vi "KB-laser dealwith.vi"(0 "Image  input":T1(plugin-control), 1 "Image  input  copy":T1(plugin-control), 3 "Src Data 过滤0":dbl[][](array[numeric]), 4 "Src Data 过滤3.2":dbl[][](array[numeric]), 5 "Row Select Laser":string(combo)="Item4", 6 "Param List Laser Input":string[][](table), 7 "y":dbl=200.0 format="%#_13g", 8 "数值 2":dbl=0.5 format="%#_13g", 9 "raoto1":dbl=0.8 format="%#_13g") -> (11 "外环3D":dbl[][](array[numeric]), 12 "内外3D":dbl[][](array[numeric]), 13 "内环3D":dbl[][](array[numeric]), 14 "Result Array":string[](array[string]), 15 "Image Baser":T1(plugin-control), 19 "Image Baser 2":T1(plugin-control))   [LabVIEW 2015]
uses:
  <vilib>/vision/Measure.llb/Edge Options.ctl
  <vilib>/vision/Measure.llb/Edge Polarity.ctl
panel:
  out "同心度":dbl
  out "Row Select Laser 2":string(combo)="Item4"
  out "x-y":dbl
  out "矩形ROS new":string[](array[string])
  out "元素":T2 {"Contours"."Type" items=["No Selection", "Point", "Line", "Rectangle", "Oval", "Polygon", "Freehand Region", "Annulus", "Unused2", "Unused3", "Broken Line", "Freehand Line", "Rotated Rectangle"]}
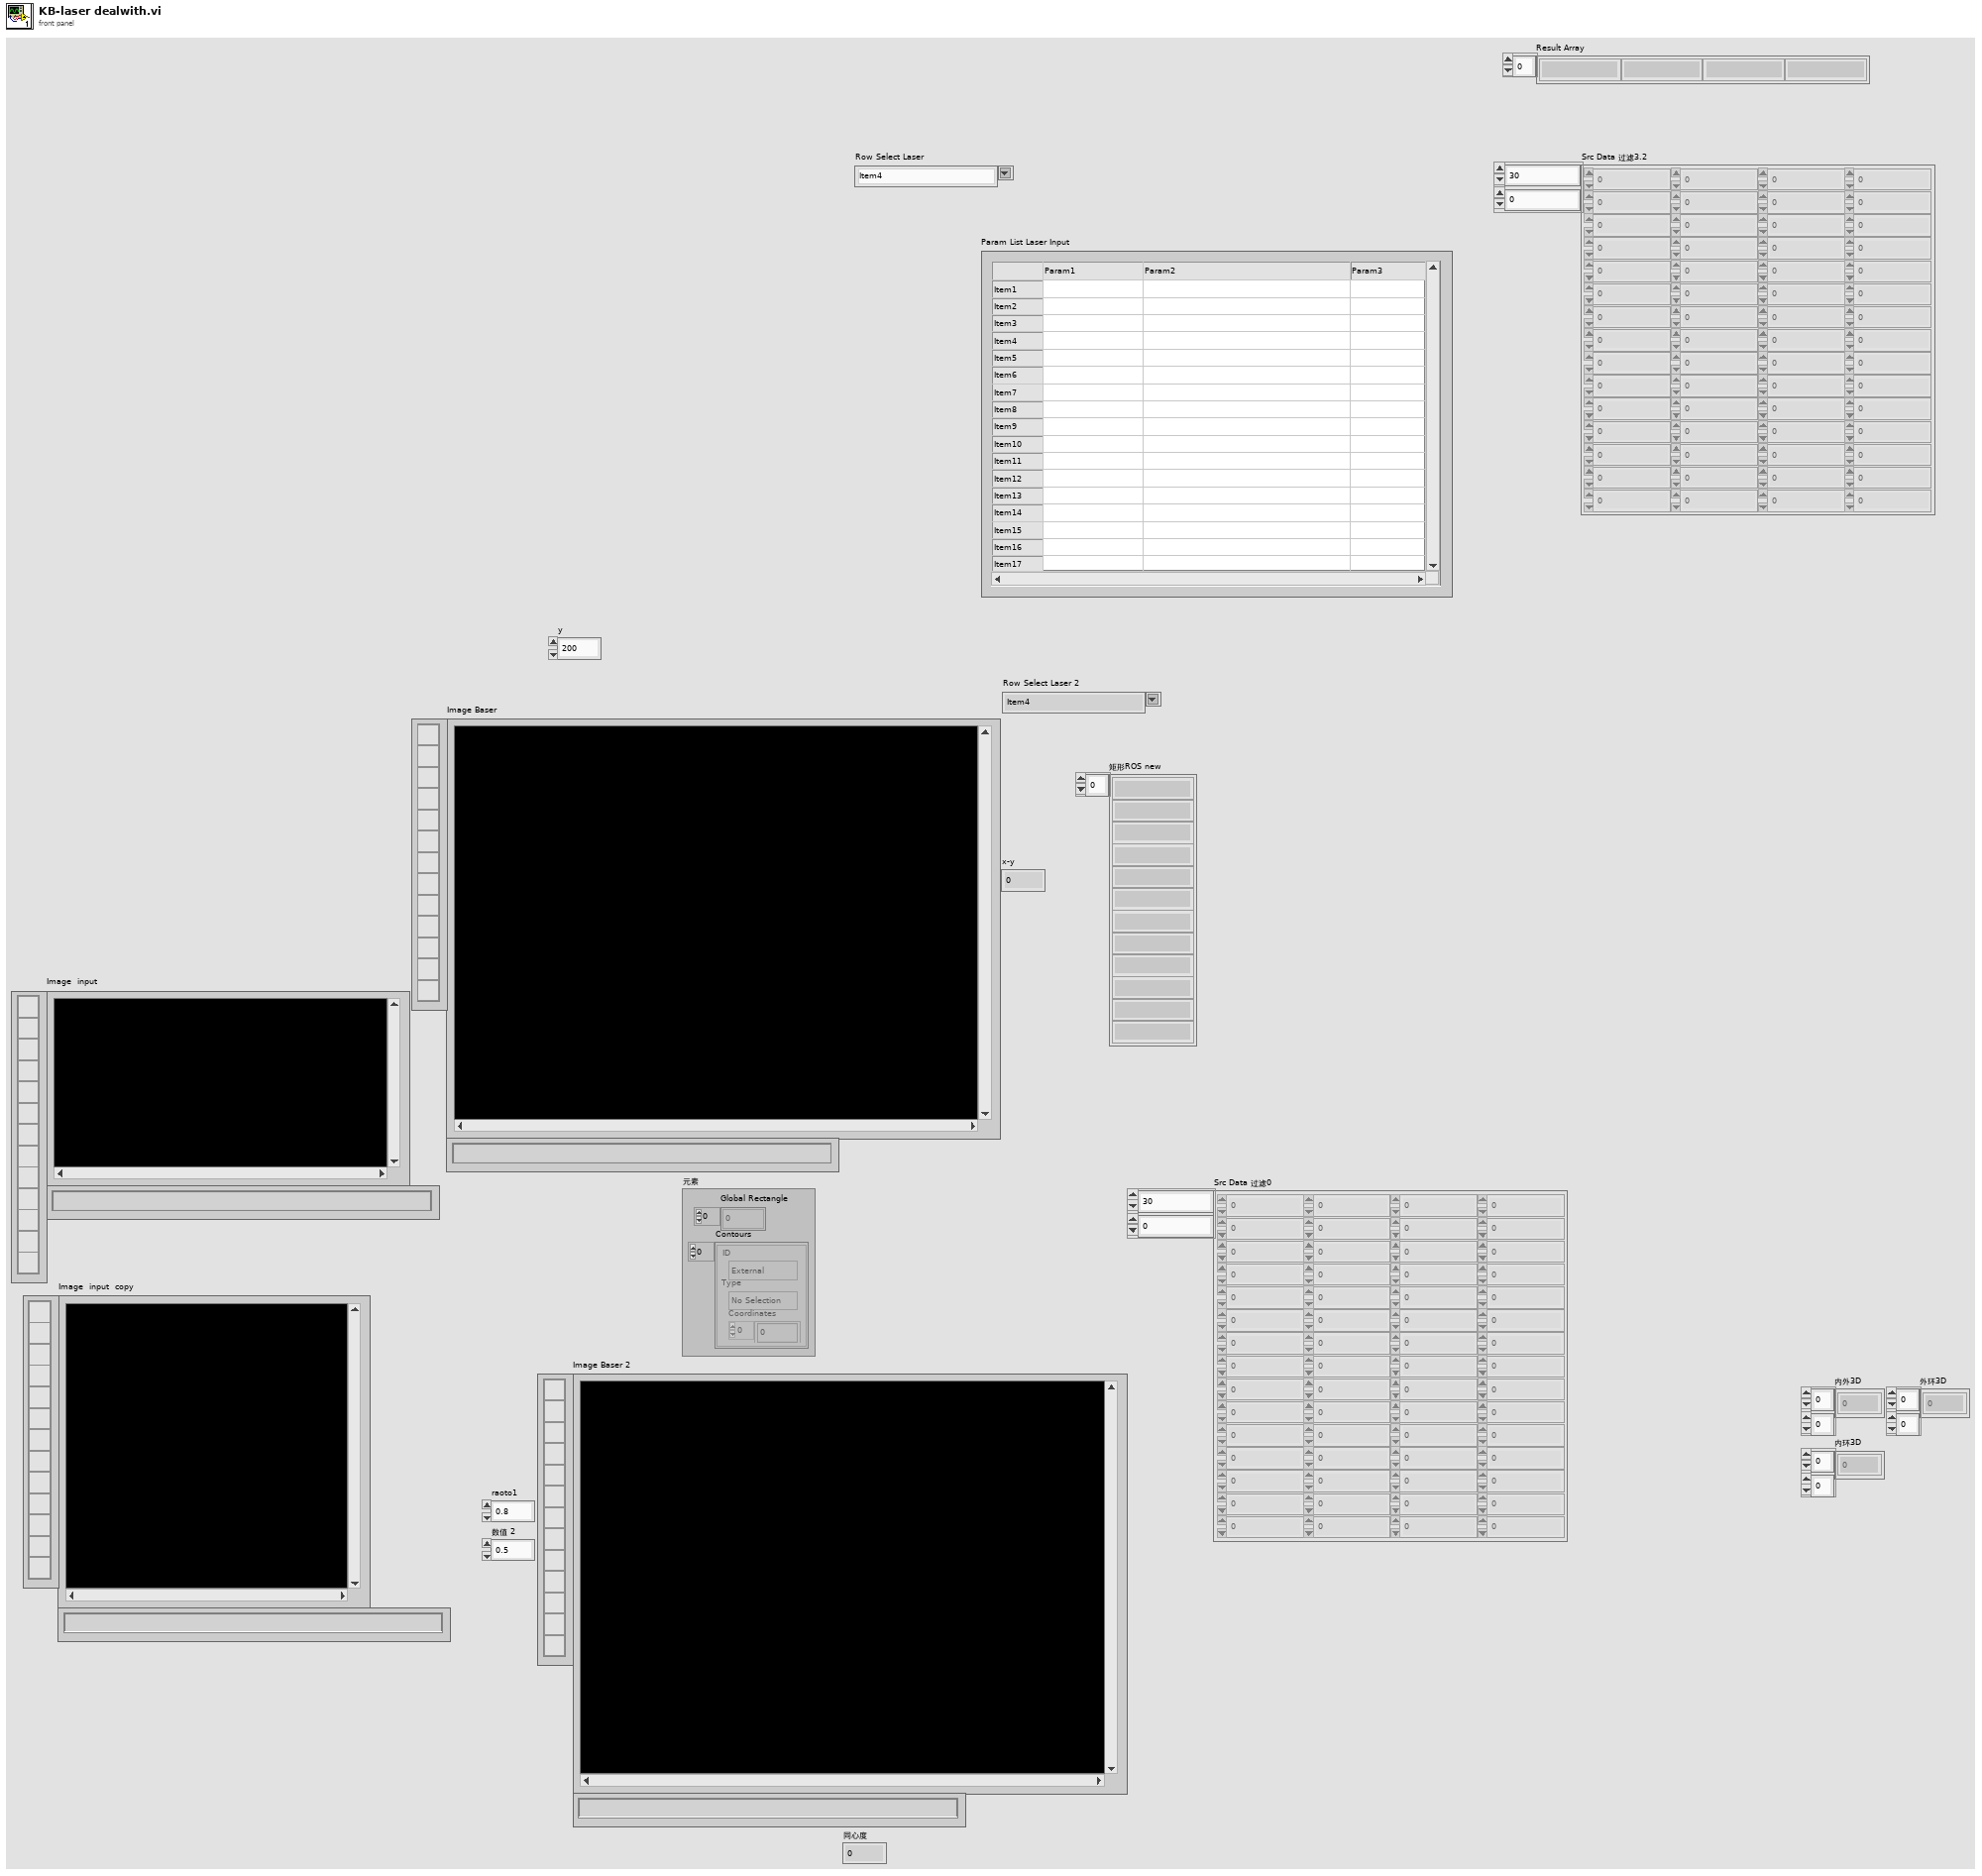
[diagram p1: front panel]
types:
  T1 = typedef "IMAQ Image.ctl" = refnum<image>
  T2 = typedef "ROI Descriptor" = cluster{"Global Rectangle":i32[], "Contours":cluster{"ID":enum32{"External", "Internal"}, "Type":u32, "Coordinates":i32[]}[]}
  T3 = typedef "Edge Options.ctl" = cluster{"Edge Polarity":T4, "Kernel Size":u32, "Width":u32, "Minimum Edge Strength":sgl, "Interpolation Type":enum32{"Zero Order", "Bilinear", "Quadratic", "Cubic", "Bilinear Fixed"}, "Data Processing Method":enum32{"Average", "Median"}}
  T4 = typedef "Edge Polarity.ctl" = u32
  T5 = cluster{"Search  Direction":u32, "Edge Options":T3, "Show Search Area":bool, "Show Search Lines":bool, "Show Edges Found":bool, "Show Result":bool, "Search Area Color":u32, "Search Lines Color":u32, "Edge Locations Color":u32, "Result Color":u32, "Overlay Group Name":string}
  T6 = cluster{"Center (Pixels)":cluster{"X":sgl, "Y":sgl}, "Radius (Pixels)":dbl, "Center (Real-World)":cluster{"X":sgl, "Y":sgl}, "Radius (Real-World)":dbl, "Roundness (Real-World)":dbl, "Average Strength":dbl, "Average SNR (dB)":dbl}
  T7 = typedef "IMAQ GM Match Report.ctl" = cluster{"Position":cluster{"x":sgl, "y":sgl}, "Angle":sgl, "Scale":sgl, "Score":sgl, "Bounding Box":cluster{"x":sgl, "y":sgl}[], "Contrast Reversed":bool, "Occlusion %":sgl, "Template Target Curve Score":sgl, "Target Template Curve Score":sgl, "Correlation Score":sgl}
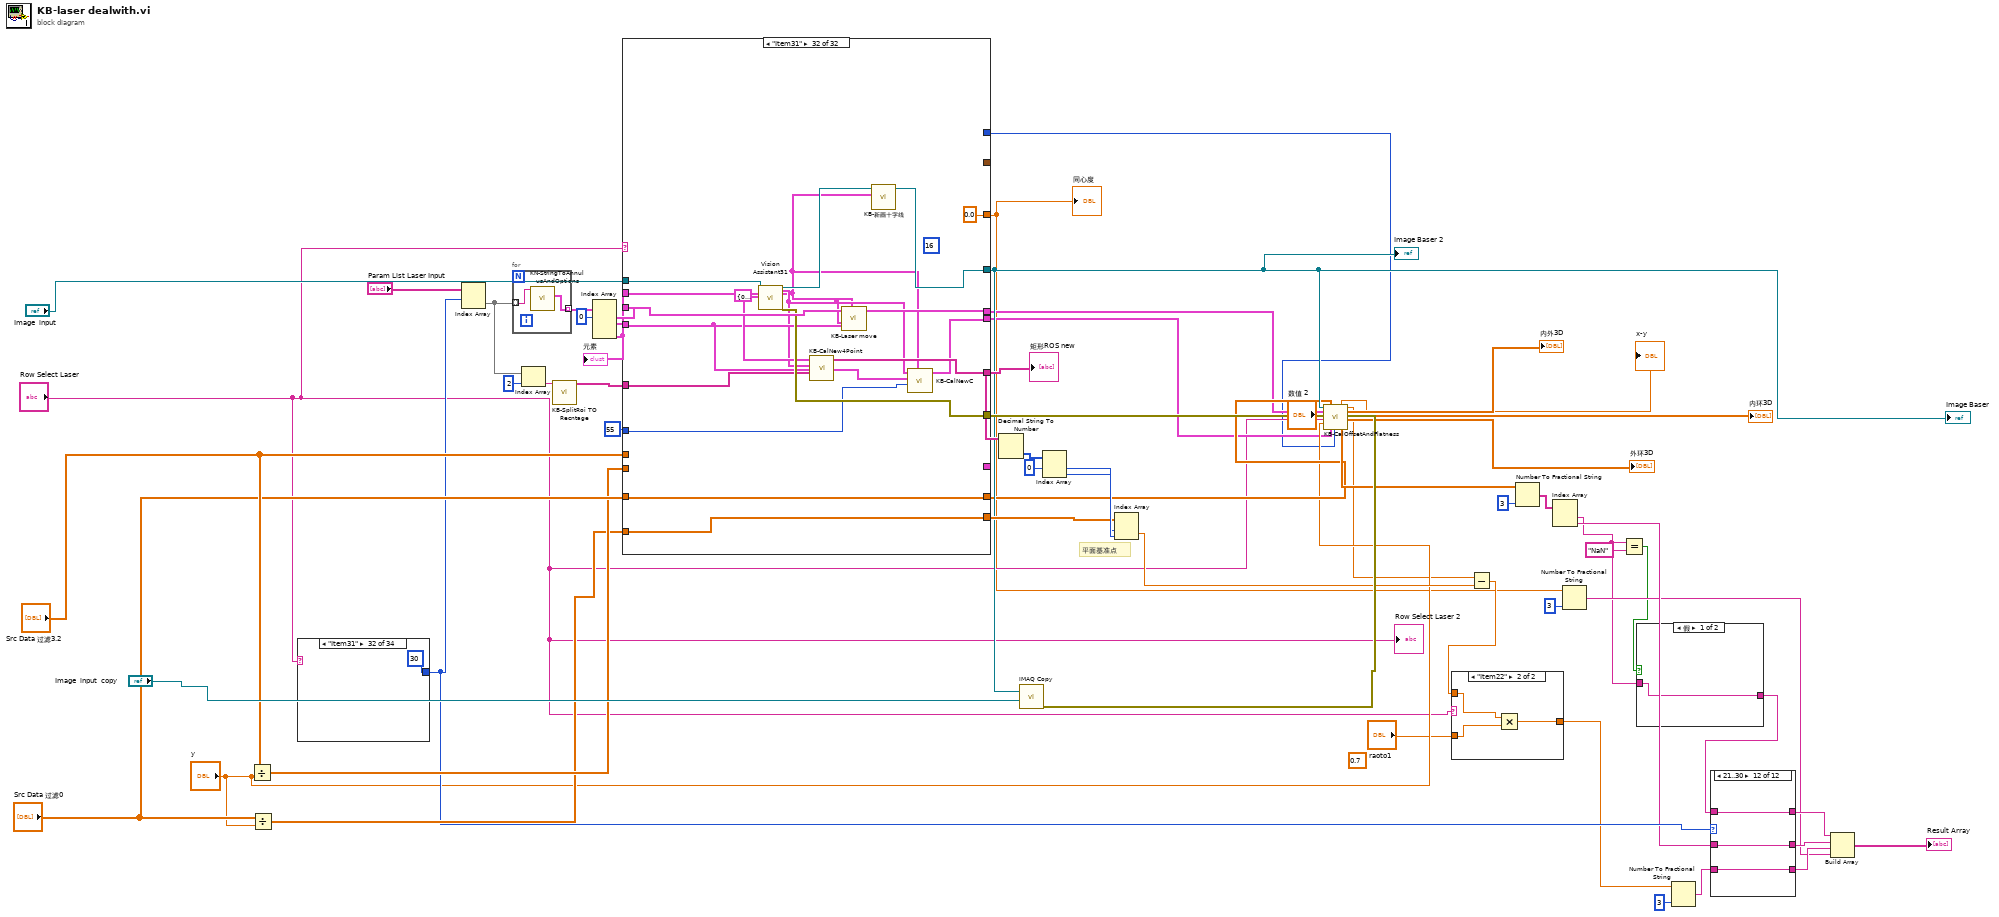
[diagram p0: block diagram]
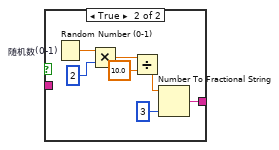
[diagram p2: hidden frame]
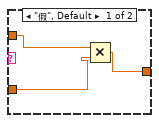
[diagram p3: hidden frame]
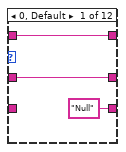
[diagram p4: hidden frame]
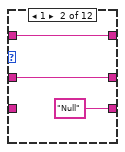
[diagram p5: hidden frame]
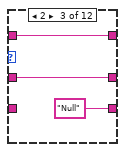
[diagram p6: hidden frame]
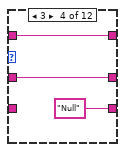
[diagram p7: hidden frame]
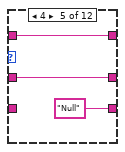
[diagram p8: hidden frame]
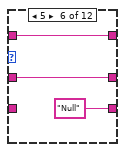
[diagram p9: hidden frame]
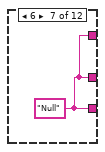
[diagram p10: hidden frame]
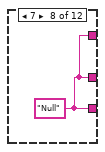
[diagram p11: hidden frame]
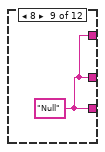
[diagram p12: hidden frame]
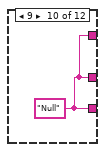
[diagram p13: hidden frame]
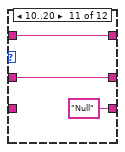
[diagram p14: hidden frame]
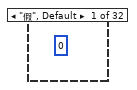
[diagram p15: hidden frame]
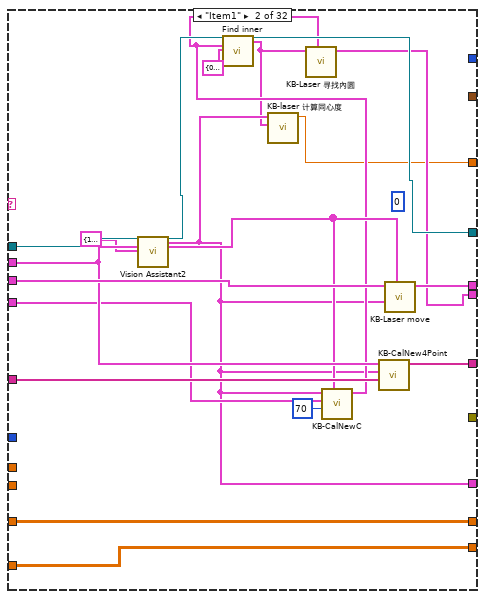
[diagram p16: hidden frame]
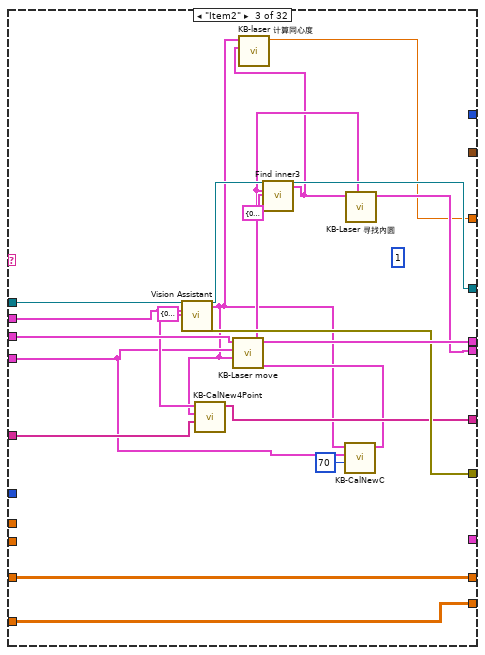
[diagram p17: hidden frame]
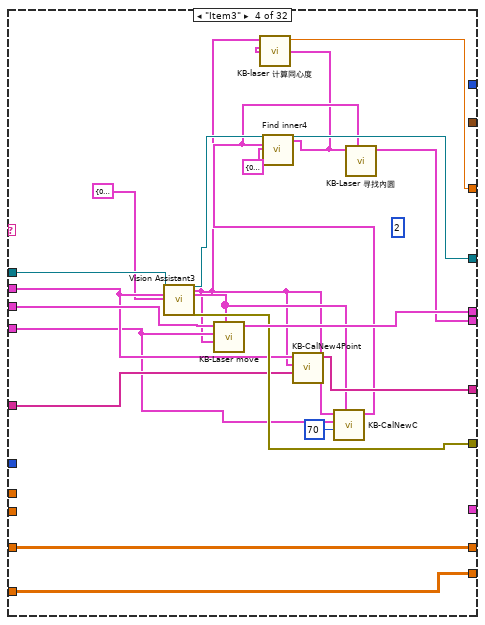
[diagram p18: hidden frame]
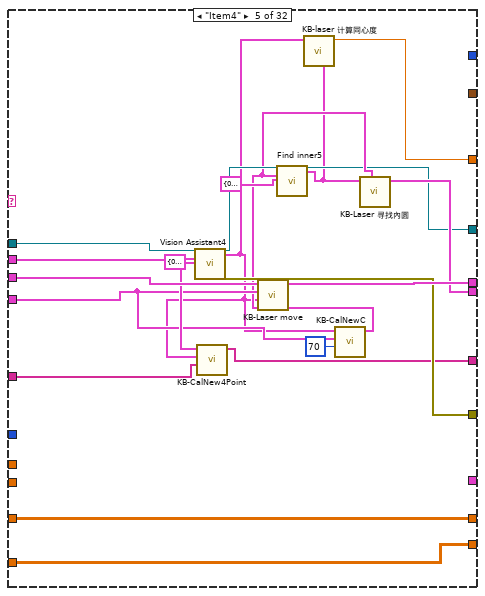
[diagram p19: hidden frame]
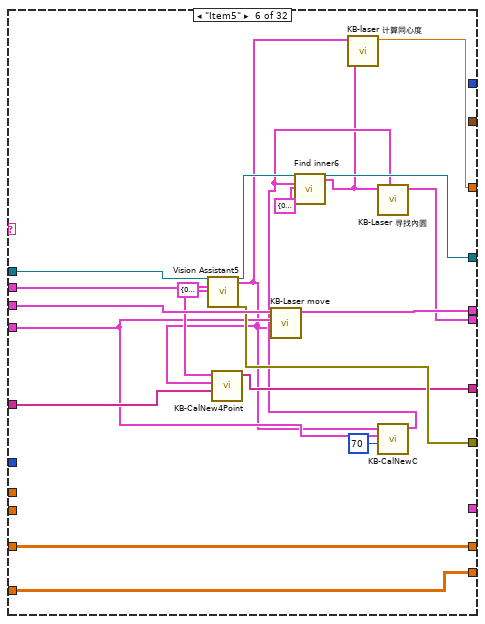
[diagram p20: hidden frame]
diagram:
  (unwired) 0.7 ("y")
  # "平面基准点"
  n1 = Divide(x="Src Data 过滤3.2", y="y") -> (x/y=w43:dbl[][])
  n2 = Divide(x="Src Data 过滤0", y="y") -> (x/y=w42:dbl[][])
  n3 = case shown="\"Item31\"" "Row Select Laser" {
    tunnel: [0 0 1 2 3 4 5 6 7 8 9 10 11 12 13 14 15 16 17 18 19 20 21 22 23 24 25 26 27 28 29 30 31 32] -> w41
    frame "假", Default {
    }
    frame "Item1" {
    }
    frame "Item2" {
    }
    frame "Item3" {
    }
    frame "Item4" {
    }
    frame "Item5" {
    }
    frame "Item6" {
    }
    frame "Item7" {
    }
    frame "Item8" {
    }
    frame "Item9" {
    }
    frame "Item10" {
    }
    frame "Item11" {
    }
    frame "Item12" {
    }
    frame "Item13" {
    }
    frame "Item14" {
    }
    frame "Item15" {
    }
    frame "Item16" {
    }
    frame "Item17" {
    }
    frame "Item18" {
    }
    frame "Item19" {
    }
    frame "Item20" {
    }
    frame "Item21" {
    }
    frame "Item22" {
    }
    frame "Item23" {
    }
    frame "Item24" {
    }
    frame "Item25" {
    }
    frame "Item26" {
    }
    frame "Item27" {
    }
    frame "Item28" {
    }
    frame "Item29" {
    }
    frame "Item30" {
    }
    frame "Item31" {
    }
    frame "Item32" {
    }
    frame "Item33" {
    }
  }
  n4 = Index Array(array="Param List Laser Input", index (row)=w41) -> (element=w54:string[])  [unwired: 1 in]
  n5 = for {
    tunnel: w54 -> [w95] mode=indexing
    tunnel: [w94] -> w58 mode=indexing
    n6 = call "KN-StringToAnnulusAndOptions.vi"("String"=w95) -> ("ROI Descriptor"=w94:T2)  [unwired: 5 in, 5 out]
  }
  n7 = Index Array(array=w54, index=2 ("索引")) -> (element=w52:string)
  n8 = call "KB-SplitRoi TO Recntage.vi"("String 2"=w52) -> ("数组"=w47:string[])  [unwired: 10 in]
  n9 = Index Array(array=w58, index #1=0 ("索引")) -> (element #1=w50:T2, element #2=w49:T2, element #4=w45:T2)  [unwired: 3 in, 1 out]
  "元素" <- w45
  n10 = case shown="\"Item31\"" "Row Select Laser" {
    tunnel: [_ w103 w122 w142 w160 w183 w203 w219 w233 w250 w266 w282 w301 w321 w337 w359 w377 w395 w417 w436 w455 w474 w492 w504 w521 w538 w555 w572 w589 w606 w625 w642] -> w24
    tunnel: "Image  input" -> [_ w115 w135 w156 w176 w196 w215 w229 w243 w259 w275 w294 w314 w328 w352 w372 w391 w410 w429 w448 w467 w486 w494 w517 w534 w551 w568 w585 w592 w619 w637 w655]
    tunnel: w45 -> [_ w112 w131 w152 w172 w192 w212 w226 w240 w256 w272 w291 w311 w327 w349 w369 w388 w407 w426 w445 w464 w483 w493 w514 w531 w548 w565 w582 w600 w616 w634 w651]
    tunnel: w50 -> [_ w114 w134 w155 w175 w195 w214 w228 w242 w258 w274 w293 w313 w333 w351 w371 w390 w409 w428 w447 w466 w485 w502 w516 w533 w550 w567 w584 w602 w618 w636 w654]
    tunnel: w49 -> [_ w102 w128 w149 w169 w189 w209 w223 w237 w249 w265 w288 w308 w329 w346 w366 w385 w404 w423 w442 w461 w480 w499 w511 w528 w545 w562 w579 w597 w613 w631 w648]
    tunnel: [_ w113 w133 w154 w174 w194 w213 w227 w241 w257 w273 w292 w312 w332 w350 w370 w389 w408 w427 w446 w465 w484 w501 w515 w532 w549 w566 w583 w601 w617 w635 w653] -> w22
    tunnel: [_ w100 w120 w140 w162 w181 w201 w222 w236 w248 w264 w280 w299 w319 w339 w357 w378 w397 w415 w434 w453 w472 w498 w510 w527 w544 w561 w578 w596 w612 w630 w647] -> w20
    tunnel: [_ _ w132 w153 w173 w193 _ _ _ _ _ _ _ _ _ _ _ _ _ _ _ _ _ _ _ _ _ _ _ _ _ w652] -> w48
    tunnel: w47 -> [_ w110 w130 w151 w171 w191 w211 w225 w239 w254 w270 w290 w310 w331 w348 w368 w387 w406 w425 w444 w463 w482 w497 w513 w530 w547 w564 w581 w599 w615 w633 w650]
    tunnel: [_ w111 w129 w150 w170 w190 w210 w224 w238 w253 w269 w289 w309 w330 w347 w367 w386 w405 w424 w443 w462 w481 w500 w512 w529 w546 w563 w580 w598 w614 w632 w649] -> w33
    tunnel: "Src Data 过滤3.2" -> [_ _ _ _ _ _ _ _ _ _ _ _ _ _ _ _ _ _ _ _ _ _ _ _ _ _ _ _ _ _ _ _]
    tunnel: "Src Data 过滤0" -> [_ w108 w126 w147 w168 w188 w208 w221 w235 w247 w263 w287 w307 w326 w344 w364 w384 w403 w422 w441 w460 w479 w496 w509 w526 w543 w560 w577 w595 w611 w629 w646]
    tunnel: [_ w108 w126 w147 w168 w188 w208 w221 w235 w247 w263 w287 w307 w326 w344 w364 w384 w403 w422 w441 w460 w479 w496 w509 w526 w543 w560 w577 w595 w611 w629 w646] -> w23
    tunnel: [_ w109 w127 w148 w167 w187 w207 w220 w234 w246 w262 w286 w306 w325 w345 w365 w383 w402 w421 w440 w459 w478 w495 w508 w525 w542 w559 w576 w594 w610 w628 w645] -> w25
    tunnel: w43 -> [_ _ _ _ _ _ _ _ _ _ _ _ _ _ _ _ _ _ _ _ _ _ _ _ _ _ _ _ _ _ _ _]
    tunnel: w42 -> [_ w109 w127 w148 w167 w187 w207 w220 w234 w246 w262 w286 w306 w325 w345 w365 w383 w402 w421 w440 w459 w478 w495 w508 w525 w542 w559 w576 w594 w610 w628 w645]
    tunnel: [_ w98 _ _ _ _ _ _ _ _ _ _ _ _ _ _ _ _ _ _ _ _ _ _ _ _ _ _ _ _ _ _] -> _
    tunnel: 55 ("Outer Radius") -> [_ _ _ _ _ _ _ w217 w231 w245 w261 _ _ _ _ _ _ _ _ _ _ _ _ w506 w523 w540 w557 w574 w591 w608 w627 w640]
    tunnel: [_ _ _ _ _ _ _ _ _ _ _ _ _ _ _ _ _ _ _ _ _ _ _ _ _ _ _ _ _ _ w622 _] -> _
    tunnel: [_ w96 w116 w136 w157 w177 w197 0.0 ("Radius (Real-World)") 0.0 ("Radius (Real-World)") 0.0 ("Radius (Real-World)") 0.0 ("Radius (Real-World)") w276 w295 w315 w334 w353 w373 w392 w411 w430 w449 w468 0.0 ("Radius (Real-World)") 0.0 ("Radius (Real-World)") 0.0 ("Radius (Real-World)") 0.0 ("Radius (Real-World)") 0.0 ("Radius (Real-World)") 0.0 ("Radius (Real-World)") 0.0 ("Radius (Real-World)") 0.0 ("Radius (Real-World)") 0.0 ("Radius (Real-World)") 0.0 ("Radius (Real-World)")] -> w8
    tunnel: [_ _ _ _ _ _ _ _ _ _ _ _ _ _ _ _ _ _ _ _ _ _ 22 _ _ _ _ _ _ _ _ _] -> w10
    frame "假", Default {
      (unwired) 0
    }
    frame "Item1" {
      (unwired) 0
      n11 = call "Vision Assistant2"("Image In"=w115, "ROI Descriptor (Find Circular Edge 1)"=w112, "Options (Find Circular Edge 1)"=T5 {"Search  Direction"=1, "Edge Options"={"Edge Polarity"=2, "Kernel Size"=3, "Width"=3, "Minimum Edge Strength"=38.0, "Interpolation Type"=enum."Bilinear Fixed", "Data Processing Method"=enum."Average"}, "Show Search Area"=TRUE, "Show Search Lines"=FALSE, "Show Edges Found"=FALSE, "Show Result"=TRUE, "Search Area Color"=65280, "Search Lines Color"=255, "Edge Locations Color"=16776960, "Result Color"=16711680, "Overlay Group Name"=""}) -> ("Image Out"=w105:T1, "Fitted Circle (Find Circular Edge 1)"=w98:T6, "Matches (Geometric Matching 1)"=w107:T7[])  [unwired: 21 in, 1 out]
      n12 = call "KB-CalNewC.vi"("Matches (Geometric Matching 1)"=w107, "Outer Radius"=70, "I roi"=w102, "Fitted Circle (Find Circular Edge 1)"=w98) -> ("ROI Descriptor"=w101:T2)  [unwired: 7 in]
      n13 = call "Find inner"("Image In"=w105, "ROI Descriptor (Find Circular Edge 1)"=w101, "Options (Find Circular Edge 1)"=T5 {"Search  Direction"=0, "Edge Options"={"Edge Polarity"=2, "Kernel Size"=3, "Width"=3, "Minimum Edge Strength"=1.0, "Interpolation Type"=enum."Bilinear Fixed", "Data Processing Method"=enum."Average"}, "Show Search Area"=TRUE, "Show Search Lines"=FALSE, "Show Edges Found"=FALSE, "Show Result"=TRUE, "Search Area Color"=65280, "Search Lines Color"=255, "Edge Locations Color"=16776960, "Result Color"=16711680, "Overlay Group Name"=""}) -> ("Image Out"=w103:T1, "Fitted Circle (Find Circular Edge 1)"=w97:T6)  [unwired: 22 in, 1 out]
      n14 = call "KB-laser 计算同心度.vi"("小圆圆心"=w97, "大圆圆心"=w98) -> ("sqrt(x)"=w96:sgl)  [unwired: 9 in]
      n15 = call "KB-Laser 寻找內圆.vi"("旧ROI"=w101, "新圆心"=w97) -> ("ROI Descriptor"=w100:T2)  [unwired: 6 in, 3 out]
      n16 = call "KB-CalNew4Point.vi"("矩形ROS 原始"=w110, "Fitted Circle (Find Circular Edge 1) New"=w98, "原始寻心点"=w112) -> ("矩形ROS new"=w111:string[])  [unwired: 8 in]
      n17 = call "KB-Laser move.vi"("Matches (Geometric Matching 1)"=w107, "Fitted Circle (Find Circular Edge 1)"=w98, "O roi"=w114) -> ("O roi Out"=w113:T2)  [unwired: 7 in, 1 out]
    }
    frame "Item2" {
      (unwired) 1
      n18 = call "Vision Assistant"("Image In"=w135, "ROI Descriptor (Find Circular Edge 1)"=w131, "Options (Find Circular Edge 1)"=T5 {"Search  Direction"=0, "Edge Options"={"Edge Polarity"=1, "Kernel Size"=3, "Width"=3, "Minimum Edge Strength"=30.0, "Interpolation Type"=enum."Bilinear Fixed", "Data Processing Method"=enum."Average"}, "Show Search Area"=TRUE, "Show Search Lines"=FALSE, "Show Edges Found"=FALSE, "Show Result"=TRUE, "Search Area Color"=65280, "Search Lines Color"=255, "Edge Locations Color"=16776960, "Result Color"=16711680, "Overlay Group Name"=""}) -> ("Image Out"=w123:T1, "Fitted Circle (Find Circular Edge 1)"=w118:T6, "error out"=w132:errorcluster)  [unwired: 21 in, 1 out]
      n19 = call "KB-CalNew4Point.vi"("矩形ROS 原始"=w130, "Fitted Circle (Find Circular Edge 1) New"=w118, "原始寻心点"=w131) -> ("矩形ROS new"=w129:string[])  [unwired: 8 in]
      n20 = call "KB-Laser move.vi"("Fitted Circle (Find Circular Edge 1)"=w118, "I roi"=w128, "O roi"=w134) -> ("O roi Out"=w133:T2)  [unwired: 7 in, 1 out]
      n21 = call "KB-CalNewC.vi"("Outer Radius"=70, "I roi"=w128, "Fitted Circle (Find Circular Edge 1)"=w118) -> ("ROI Descriptor"=w121:T2)  [unwired: 8 in]
      n22 = call "Find inner3"("Image In"=w123, "ROI Descriptor (Find Circular Edge 1)"=w121, "Options (Find Circular Edge 1)"=T5 {"Search  Direction"=0, "Edge Options"={"Edge Polarity"=2, "Kernel Size"=3, "Width"=3, "Minimum Edge Strength"=1.0, "Interpolation Type"=enum."Bilinear Fixed", "Data Processing Method"=enum."Average"}, "Show Search Area"=TRUE, "Show Search Lines"=FALSE, "Show Edges Found"=FALSE, "Show Result"=TRUE, "Search Area Color"=65280, "Search Lines Color"=255, "Edge Locations Color"=16776960, "Result Color"=16711680, "Overlay Group Name"=""}) -> ("Image Out"=w122:T1, "Fitted Circle (Find Circular Edge 1)"=w117:T6)  [unwired: 22 in, 1 out]
      n23 = call "KB-laser 计算同心度.vi"("小圆圆心"=w117, "大圆圆心"=w118) -> ("sqrt(x)"=w116:sgl)  [unwired: 9 in]
      n24 = call "KB-Laser 寻找內圆.vi"("旧ROI"=w121, "新圆心"=w117) -> ("ROI Descriptor"=w120:T2)  [unwired: 6 in, 3 out]
    }
    frame "Item3" {
      (unwired) 2
      n25 = call "Vision Assistant3"("Image In"=w156, "ROI Descriptor (Find Circular Edge 1)"=w152, "Options (Find Circular Edge 1)"=T5 {"Search  Direction"=0, "Edge Options"={"Edge Polarity"=1, "Kernel Size"=13, "Width"=13, "Minimum Edge Strength"=35.0, "Interpolation Type"=enum."Bilinear Fixed", "Data Processing Method"=enum."Average"}, "Show Search Area"=TRUE, "Show Search Lines"=FALSE, "Show Edges Found"=FALSE, "Show Result"=TRUE, "Search Area Color"=65280, "Search Lines Color"=255, "Edge Locations Color"=16776960, "Result Color"=16711680, "Overlay Group Name"=""}) -> ("Image Out"=w143:T1, "Fitted Circle (Find Circular Edge 1)"=w138:T6, "Matches (Geometric Matching 1)"=w146:T7[], "error out"=w153:errorcluster)  [unwired: 21 in]
      n26 = call "KB-Laser move.vi"("Matches (Geometric Matching 1)"=w146, "Fitted Circle (Find Circular Edge 1)"=w138, "I roi"=w149, "O roi"=w155) -> ("O roi Out"=w154:T2)  [unwired: 6 in, 1 out]
      n27 = call "KB-CalNew4Point.vi"("矩形ROS 原始"=w151, "Fitted Circle (Find Circular Edge 1) New"=w138, "原始寻心点"=w152) -> ("矩形ROS new"=w150:string[])  [unwired: 8 in]
      n28 = call "KB-CalNewC.vi"("Matches (Geometric Matching 1)"=w146, "Outer Radius"=70, "I roi"=w149, "Fitted Circle (Find Circular Edge 1)"=w138) -> ("ROI Descriptor"=w141:T2)  [unwired: 7 in]
      n29 = call "Find inner4"("Image In"=w143, "ROI Descriptor (Find Circular Edge 1)"=w141, "Options (Find Circular Edge 1)"=T5 {"Search  Direction"=0, "Edge Options"={"Edge Polarity"=2, "Kernel Size"=3, "Width"=3, "Minimum Edge Strength"=1.0, "Interpolation Type"=enum."Bilinear Fixed", "Data Processing Method"=enum."Average"}, "Show Search Area"=TRUE, "Show Search Lines"=FALSE, "Show Edges Found"=FALSE, "Show Result"=TRUE, "Search Area Color"=65280, "Search Lines Color"=255, "Edge Locations Color"=16776960, "Result Color"=16711680, "Overlay Group Name"=""}) -> ("Image Out"=w142:T1, "Fitted Circle (Find Circular Edge 1)"=w137:T6)  [unwired: 22 in, 1 out]
      n30 = call "KB-laser 计算同心度.vi"("小圆圆心"=w137, "大圆圆心"=w138) -> ("sqrt(x)"=w136:sgl)  [unwired: 9 in]
      n31 = call "KB-Laser 寻找內圆.vi"("旧ROI"=w141, "新圆心"=w137) -> ("ROI Descriptor"=w140:T2)  [unwired: 6 in, 3 out]
    }
    frame "Item4" {
      n32 = call "Vision Assistant4"("Image In"=w176, "ROI Descriptor (Find Circular Edge 1)"=w172, "Options (Find Circular Edge 1)"=T5 {"Search  Direction"=0, "Edge Options"={"Edge Polarity"=1, "Kernel Size"=3, "Width"=3, "Minimum Edge Strength"=32.0, "Interpolation Type"=enum."Bilinear Fixed", "Data Processing Method"=enum."Average"}, "Show Search Area"=TRUE, "Show Search Lines"=FALSE, "Show Edges Found"=FALSE, "Show Result"=TRUE, "Search Area Color"=65280, "Search Lines Color"=255, "Edge Locations Color"=16776960, "Result Color"=16711680, "Overlay Group Name"=""}) -> ("Image Out"=w164:T1, "Fitted Circle (Find Circular Edge 1)"=w159:T6, "error out"=w173:errorcluster)  [unwired: 21 in, 1 out]
      n33 = call "KB-CalNew4Point.vi"("矩形ROS 原始"=w171, "Fitted Circle (Find Circular Edge 1) New"=w159, "原始寻心点"=w172) -> ("矩形ROS new"=w170:string[])  [unwired: 8 in]
      n34 = call "KB-Laser move.vi"("Fitted Circle (Find Circular Edge 1)"=w159, "I roi"=w169, "O roi"=w175) -> ("O roi Out"=w174:T2)  [unwired: 7 in, 1 out]
      n35 = call "KB-CalNewC.vi"("Outer Radius"=70, "I roi"=w169, "Fitted Circle (Find Circular Edge 1)"=w159) -> ("ROI Descriptor"=w163:T2)  [unwired: 8 in]
      n36 = call "Find inner5"("Image In"=w164, "ROI Descriptor (Find Circular Edge 1)"=w163, "Options (Find Circular Edge 1)"=T5 {"Search  Direction"=0, "Edge Options"={"Edge Polarity"=2, "Kernel Size"=3, "Width"=3, "Minimum Edge Strength"=1.0, "Interpolation Type"=enum."Bilinear Fixed", "Data Processing Method"=enum."Average"}, "Show Search Area"=TRUE, "Show Search Lines"=FALSE, "Show Edges Found"=FALSE, "Show Result"=TRUE, "Search Area Color"=65280, "Search Lines Color"=255, "Edge Locations Color"=16776960, "Result Color"=16711680, "Overlay Group Name"=""}) -> ("Image Out"=w160:T1, "Fitted Circle (Find Circular Edge 1)"=w158:T6)  [unwired: 22 in, 1 out]
      n37 = call "KB-laser 计算同心度.vi"("小圆圆心"=w158, "大圆圆心"=w159) -> ("sqrt(x)"=w157:sgl)  [unwired: 9 in]
      n38 = call "KB-Laser 寻找內圆.vi"("旧ROI"=w163, "新圆心"=w158) -> ("ROI Descriptor"=w162:T2)  [unwired: 6 in, 3 out]
    }
    frame "Item5" {
      n39 = call "Vision Assistant5"("Image In"=w196, "ROI Descriptor (Find Circular Edge 1)"=w192, "Options (Find Circular Edge 1)"=T5 {"Search  Direction"=0, "Edge Options"={"Edge Polarity"=1, "Kernel Size"=3, "Width"=3, "Minimum Edge Strength"=52.0, "Interpolation Type"=enum."Bilinear Fixed", "Data Processing Method"=enum."Average"}, "Show Search Area"=TRUE, "Show Search Lines"=FALSE, "Show Edges Found"=FALSE, "Show Result"=TRUE, "Search Area Color"=65280, "Search Lines Color"=255, "Edge Locations Color"=16776960, "Result Color"=16711680, "Overlay Group Name"=""}) -> ("Image Out"=w184:T1, "Fitted Circle (Find Circular Edge 1)"=w179:T6, "error out"=w193:errorcluster)  [unwired: 21 in, 1 out]
      n40 = call "KB-CalNew4Point.vi"("矩形ROS 原始"=w191, "Fitted Circle (Find Circular Edge 1) New"=w179, "原始寻心点"=w192) -> ("矩形ROS new"=w190:string[])  [unwired: 8 in]
      n41 = call "KB-Laser move.vi"("Fitted Circle (Find Circular Edge 1)"=w179, "I roi"=w189, "O roi"=w195) -> ("O roi Out"=w194:T2)  [unwired: 7 in, 1 out]
      n42 = call "KB-CalNewC.vi"("Outer Radius"=70, "I roi"=w189, "Fitted Circle (Find Circular Edge 1)"=w179) -> ("ROI Descriptor"=w182:T2)  [unwired: 8 in]
      n43 = call "Find inner6"("Image In"=w184, "ROI Descriptor (Find Circular Edge 1)"=w182, "Options (Find Circular Edge 1)"=T5 {"Search  Direction"=0, "Edge Options"={"Edge Polarity"=2, "Kernel Size"=3, "Width"=3, "Minimum Edge Strength"=1.0, "Interpolation Type"=enum."Bilinear Fixed", "Data Processing Method"=enum."Average"}, "Show Search Area"=TRUE, "Show Search Lines"=FALSE, "Show Edges Found"=FALSE, "Show Result"=TRUE, "Search Area Color"=65280, "Search Lines Color"=255, "Edge Locations Color"=16776960, "Result Color"=16711680, "Overlay Group Name"=""}) -> ("Image Out"=w183:T1, "Fitted Circle (Find Circular Edge 1)"=w178:T6)  [unwired: 22 in, 1 out]
      n44 = call "KB-laser 计算同心度.vi"("小圆圆心"=w178, "大圆圆心"=w179) -> ("sqrt(x)"=w177:sgl)  [unwired: 9 in]
      n45 = call "KB-Laser 寻找內圆.vi"("旧ROI"=w182, "新圆心"=w178) -> ("ROI Descriptor"=w181:T2)  [unwired: 6 in, 3 out]
    }
    frame "Item6" {
      (unwired) 3
      n46 = call "Vision Assistant6"("Image In"=w215, "ROI Descriptor (Find Circular Edge 1)"=w212, "Options (Find Circular Edge 1)"=T5 {"Search  Direction"=0, "Edge Options"={"Edge Polarity"=1, "Kernel Size"=13, "Width"=13, "Minimum Edge Strength"=33.0, "Interpolation Type"=enum."Bilinear Fixed", "Data Processing Method"=enum."Average"}, "Show Search Area"=TRUE, "Show Search Lines"=FALSE, "Show Edges Found"=FALSE, "Show Result"=TRUE, "Search Area Color"=65280, "Search Lines Color"=255, "Edge Locations Color"=16776960, "Result Color"=16711680, "Overlay Group Name"=""}) -> ("Image Out"=w204:T1, "Fitted Circle (Find Circular Edge 1)"=w199:T6)  [unwired: 21 in, 2 out]
      n47 = call "KB-CalNew4Point.vi"("矩形ROS 原始"=w211, "Fitted Circle (Find Circular Edge 1) New"=w199, "原始寻心点"=w212) -> ("矩形ROS new"=w210:string[])  [unwired: 8 in]
      n48 = call "KB-Laser move.vi"("Fitted Circle (Find Circular Edge 1)"=w199, "I roi"=w209, "O roi"=w214) -> ("O roi Out"=w213:T2)  [unwired: 7 in, 1 out]
      n49 = call "KB-CalNewC.vi"("Outer Radius"=70, "I roi"=w209, "Fitted Circle (Find Circular Edge 1)"=w199) -> ("ROI Descriptor"=w202:T2)  [unwired: 8 in]
      n50 = call "Find inner7"("Image In"=w204, "ROI Descriptor (Find Circular Edge 1)"=w202, "Options (Find Circular Edge 1)"=T5 {"Search  Direction"=0, "Edge Options"={"Edge Polarity"=2, "Kernel Size"=3, "Width"=3, "Minimum Edge Strength"=1.0, "Interpolation Type"=enum."Bilinear Fixed", "Data Processing Method"=enum."Average"}, "Show Search Area"=TRUE, "Show Search Lines"=FALSE, "Show Edges Found"=FALSE, "Show Result"=TRUE, "Search Area Color"=65280, "Search Lines Color"=255, "Edge Locations Color"=16776960, "Result Color"=16711680, "Overlay Group Name"=""}) -> ("Image Out"=w203:T1, "Fitted Circle (Find Circular Edge 1)"=w198:T6)  [unwired: 22 in, 1 out]
      n51 = call "KB-laser 计算同心度.vi"("小圆圆心"=w198, "大圆圆心"=w199) -> ("sqrt(x)"=w197:sgl)  [unwired: 9 in]
      n52 = call "KB-Laser 寻找內圆.vi"("旧ROI"=w202, "新圆心"=w198) -> ("ROI Descriptor"=w201:T2)  [unwired: 6 in, 3 out]
    }
    frame "Item7" {
      (unwired) T5 {"Search  Direction"=1, "Edge Options"={"Edge Polarity"=0, "Kernel Size"=13, "Width"=13, "Minimum Edge Strength"=175.0, "Interpolation Type"=enum."Bilinear Fixed", "Data Processing Method"=enum."Average"}, "Show Search Area"=TRUE, "Show Search Lines"=TRUE, "Show Edges Found"=TRUE, "Show Result"=TRUE, "Search Area Color"=65280, "Search Lines Color"=255, "Edge Locations Color"=16776960, "Result Color"=16711680, "Overlay Group Name"=""} ("Options (Find Circular Edge 1)")
      (unwired) 3
      n53 = call "Vision Assistant7"("Image In"=w229, "ROI Descriptor (Find Circular Edge 1)"=w226) -> ("Image Out"=w219:T1, "Fitted Circle (Find Circular Edge 1)"=w218:T6)  [unwired: 23 in, 1 out]
      n54 = call "KB-CalNew4Point.vi"("矩形ROS 原始"=w225, "Fitted Circle (Find Circular Edge 1) New"=w218, "原始寻心点"=w226) -> ("矩形ROS new"=w224:string[])  [unwired: 8 in]
      n55 = call "KB-Laser move7-10.vi"("Fitted Circle (Find Circular Edge 1)"=w218, "I roi"=w223, "O roi"=w228) -> ("O roi Out"=w227:T2)  [unwired: 7 in, 1 out]
      n56 = call "KB-CalNewC.vi"("Outer Radius"=w217, "I roi"=w223, "Fitted Circle (Find Circular Edge 1)"=w218) -> ("ROI Descriptor"=w222:T2)  [unwired: 8 in]
    }
    frame "Item8" {
      (unwired) 3
      n57 = call "Vision Assistant8"("Image In"=w243, "ROI Descriptor (Find Circular Edge 1)"=w240) -> ("Image Out"=w233:T1, "Fitted Circle (Find Circular Edge 1)"=w232:T6)  [unwired: 23 in, 1 out]
      n58 = call "KB-Laser move7-10.vi"("Fitted Circle (Find Circular Edge 1)"=w232, "I roi"=w237, "O roi"=w242) -> ("O roi Out"=w241:T2)  [unwired: 7 in, 1 out]
      n59 = call "KB-CalNew4Point.vi"("矩形ROS 原始"=w239, "Fitted Circle (Find Circular Edge 1) New"=w232, "原始寻心点"=w240) -> ("矩形ROS new"=w238:string[])  [unwired: 8 in]
      n60 = call "KB-CalNewC.vi"("Outer Radius"=w231, "I roi"=w237, "Fitted Circle (Find Circular Edge 1)"=w232) -> ("ROI Descriptor"=w236:T2)  [unwired: 8 in]
    }
    frame "Item9" {
      (unwired) 3
      n61 = call "Vision Assistant9"("Image In"=w259, "ROI Descriptor (Find Circular Edge 1)"=w256) -> ("Image Out"=w251:T1, "Fitted Circle (Find Circular Edge 1)"=w255:T6)  [unwired: 23 in, 1 out]
      n62 = call "KB-CalNew4Point.vi"("矩形ROS 原始"=w254, "Fitted Circle (Find Circular Edge 1) New"=w255, "原始寻心点"=w256) -> ("矩形ROS new"=w253:string[])  [unwired: 8 in]
      n63 = call "KB-Laser move7-10.vi"("Fitted Circle (Find Circular Edge 1)"=w255, "I roi"=w249, "O roi"=w258) -> ("O roi Out"=w257:T2)  [unwired: 7 in, 1 out]
      n64 = call "Vision Assistant41"("Image In"=w251, "ROI Descriptor (Find Circular Edge 1)"=w249) -> ("Image Out"=w250:T1, "Fitted Circle (Find Circular Edge 1)"=w252:T6)  [unwired: 23 in, 1 out]
      n65 = call "KB-CalNewC.vi"("Outer Radius"=w245, "I roi"=w249, "Fitted Circle (Find Circular Edge 1)"=w252) -> ("ROI Descriptor"=w248:T2)  [unwired: 8 in]
    }
    frame "Item10" {
      (unwired) 3
      n66 = call "Vision Assistant10"("Image In"=w275, "ROI Descriptor (Find Circular Edge 1)"=w272) -> ("Image Out"=w267:T1, "Fitted Circle (Find Circular Edge 1)"=w271:T6)  [unwired: 23 in, 1 out]
      n67 = call "KB-Laser move7-10.vi"("Fitted Circle (Find Circular Edge 1)"=w271, "I roi"=w265, "O roi"=w274) -> ("O roi Out"=w273:T2)  [unwired: 7 in, 1 out]
      n68 = call "KB-CalNew4Point.vi"("矩形ROS 原始"=w270, "Fitted Circle (Find Circular Edge 1) New"=w271, "原始寻心点"=w272) -> ("矩形ROS new"=w269:string[])  [unwired: 8 in]
      n69 = call "Vision Assistant42"("Image In"=w267, "ROI Descriptor (Find Circular Edge 1)"=w265) -> ("Image Out"=w266:T1, "Fitted Circle (Find Circular Edge 1)"=w268:T6)  [unwired: 23 in, 1 out]
      n70 = call "KB-CalNewC.vi"("Outer Radius"=w261, "I roi"=w265, "Fitted Circle (Find Circular Edge 1)"=w268) -> ("ROI Descriptor"=w264:T2)  [unwired: 8 in]
    }
    frame "Item11" {
      (unwired) 3
      n71 = call "Vision Assistant11"("Image In"=w294, "ROI Descriptor (Find Circular Edge 1)"=w291, "Options (Find Circular Edge 1)"=T5 {"Search  Direction"=0, "Edge Options"={"Edge Polarity"=1, "Kernel Size"=13, "Width"=13, "Minimum Edge Strength"=35.0, "Interpolation Type"=enum."Bilinear Fixed", "Data Processing Method"=enum."Average"}, "Show Search Area"=TRUE, "Show Search Lines"=FALSE, "Show Edges Found"=FALSE, "Show Result"=TRUE, "Search Area Color"=65280, "Search Lines Color"=255, "Edge Locations Color"=16776960, "Result Color"=16711680, "Overlay Group Name"=""}) -> ("Image Out"=w283:T1, "Fitted Circle (Find Circular Edge 1)"=w278:T6)  [unwired: 21 in, 2 out]
      n72 = call "KB-Laser move.vi"("Fitted Circle (Find Circular Edge 1)"=w278, "I roi"=w288, "O roi"=w293) -> ("O roi Out"=w292:T2)  [unwired: 7 in, 1 out]
      n73 = call "KB-CalNew4Point.vi"("矩形ROS 原始"=w290, "Fitted Circle (Find Circular Edge 1) New"=w278, "原始寻心点"=w291) -> ("矩形ROS new"=w289:string[])  [unwired: 8 in]
      n74 = call "KB-CalNewC.vi"("Outer Radius"=75, "I roi"=w288, "Fitted Circle (Find Circular Edge 1)"=w278) -> ("ROI Descriptor"=w281:T2)  [unwired: 8 in]
      n75 = call "Find inner8"("Image In"=w283, "ROI Descriptor (Find Circular Edge 1)"=w281, "Options (Find Circular Edge 1)"=T5 {"Search  Direction"=0, "Edge Options"={"Edge Polarity"=2, "Kernel Size"=3, "Width"=3, "Minimum Edge Strength"=1.0, "Interpolation Type"=enum."Bilinear Fixed", "Data Processing Method"=enum."Average"}, "Show Search Area"=TRUE, "Show Search Lines"=FALSE, "Show Edges Found"=FALSE, "Show Result"=TRUE, "Search Area Color"=65280, "Search Lines Color"=255, "Edge Locations Color"=16776960, "Result Color"=16711680, "Overlay Group Name"=""}) -> ("Image Out"=w282:T1, "Fitted Circle (Find Circular Edge 1)"=w277:T6)  [unwired: 22 in, 1 out]
      n76 = call "KB-laser 计算同心度.vi"("小圆圆心"=w277, "大圆圆心"=w278) -> ("sqrt(x)"=w276:sgl)  [unwired: 9 in]
      n77 = call "KB-Laser 寻找內圆.vi"("旧ROI"=w281, "新圆心"=w277) -> ("ROI Descriptor"=w280:T2)  [unwired: 6 in, 3 out]
    }
    frame "Item12" {
      (unwired) 3
      n78 = call "Vision Assistant12"("Image In"=w314, "ROI Descriptor (Find Circular Edge 1)"=w311, "Options (Find Circular Edge 1)"=T5 {"Search  Direction"=0, "Edge Options"={"Edge Polarity"=1, "Kernel Size"=13, "Width"=13, "Minimum Edge Strength"=35.0, "Interpolation Type"=enum."Bilinear Fixed", "Data Processing Method"=enum."Average"}, "Show Search Area"=TRUE, "Show Search Lines"=FALSE, "Show Edges Found"=FALSE, "Show Result"=TRUE, "Search Area Color"=65280, "Search Lines Color"=255, "Edge Locations Color"=16776960, "Result Color"=16711680, "Overlay Group Name"=""}) -> ("Image Out"=w302:T1, "Fitted Circle (Find Circular Edge 1)"=w297:T6, "Matches (Geometric Matching 1)"=w305:T7[])  [unwired: 21 in, 1 out]
      n79 = call "KB-CalNew4Point.vi"("矩形ROS 原始"=w310, "Fitted Circle (Find Circular Edge 1) New"=w297, "原始寻心点"=w311) -> ("矩形ROS new"=w309:string[])  [unwired: 8 in]
      n80 = call "KB-Laser move.vi"("Matches (Geometric Matching 1)"=w305, "Fitted Circle (Find Circular Edge 1)"=w297, "I roi"=w308, "O roi"=w313) -> ("O roi Out"=w312:T2)  [unwired: 6 in, 1 out]
      n81 = call "KB-CalNewC.vi"("Matches (Geometric Matching 1)"=w305, "Outer Radius"=75, "I roi"=w308, "Fitted Circle (Find Circular Edge 1)"=w297) -> ("ROI Descriptor"=w300:T2)  [unwired: 7 in]
      n82 = call "Find inner9"("Image In"=w302, "ROI Descriptor (Find Circular Edge 1)"=w300, "Options (Find Circular Edge 1)"=T5 {"Search  Direction"=0, "Edge Options"={"Edge Polarity"=2, "Kernel Size"=3, "Width"=3, "Minimum Edge Strength"=1.0, "Interpolation Type"=enum."Bilinear Fixed", "Data Processing Method"=enum."Average"}, "Show Search Area"=TRUE, "Show Search Lines"=FALSE, "Show Edges Found"=FALSE, "Show Result"=TRUE, "Search Area Color"=65280, "Search Lines Color"=255, "Edge Locations Color"=16776960, "Result Color"=16711680, "Overlay Group Name"=""}) -> ("Image Out"=w301:T1, "Fitted Circle (Find Circular Edge 1)"=w296:T6)  [unwired: 22 in, 1 out]
      n83 = call "KB-laser 计算同心度.vi"("小圆圆心"=w296, "大圆圆心"=w297) -> ("sqrt(x)"=w295:sgl)  [unwired: 9 in]
      n84 = call "KB-Laser 寻找內圆.vi"("旧ROI"=w300, "新圆心"=w296) -> ("ROI Descriptor"=w299:T2)  [unwired: 6 in, 3 out]
    }
    frame "Item13" {
      (unwired) 3
      n85 = call "Vision Assistant65"("Image In"=w328, "ROI Descriptor (Find Circular Edge 1)"=w327, "Options (Find Circular Edge 1)"=T5 {"Search  Direction"=0, "Edge Options"={"Edge Polarity"=1, "Kernel Size"=13, "Width"=13, "Minimum Edge Strength"=35.0, "Interpolation Type"=enum."Bilinear Fixed", "Data Processing Method"=enum."Average"}, "Show Search Area"=TRUE, "Show Search Lines"=FALSE, "Show Edges Found"=FALSE, "Show Result"=TRUE, "Search Area Color"=65280, "Search Lines Color"=255, "Edge Locations Color"=16776960, "Result Color"=16711680, "Overlay Group Name"=""}) -> ("Image Out"=w322:T1, "Fitted Circle (Find Circular Edge 1)"=w317:T6)  [unwired: 21 in, 2 out]
      n86 = call "KB-CalNew4Point.vi"("矩形ROS 原始"=w331, "Fitted Circle (Find Circular Edge 1) New"=w317, "原始寻心点"=w327) -> ("矩形ROS new"=w330:string[])  [unwired: 8 in]
      n87 = call "KB-Laser move.vi"("Fitted Circle (Find Circular Edge 1)"=w317, "I roi"=w329, "O roi"=w333) -> ("O roi Out"=w332:T2)  [unwired: 7 in, 1 out]
      n88 = call "KB-CalNewC.vi"("Outer Radius"=75, "I roi"=w329, "Fitted Circle (Find Circular Edge 1)"=w317) -> ("ROI Descriptor"=w320:T2)  [unwired: 8 in]
      n89 = call "Find inner10"("Image In"=w322, "ROI Descriptor (Find Circular Edge 1)"=w320, "Options (Find Circular Edge 1)"=T5 {"Search  Direction"=0, "Edge Options"={"Edge Polarity"=2, "Kernel Size"=3, "Width"=3, "Minimum Edge Strength"=1.0, "Interpolation Type"=enum."Bilinear Fixed", "Data Processing Method"=enum."Average"}, "Show Search Area"=TRUE, "Show Search Lines"=FALSE, "Show Edges Found"=FALSE, "Show Result"=TRUE, "Search Area Color"=65280, "Search Lines Color"=255, "Edge Locations Color"=16776960, "Result Color"=16711680, "Overlay Group Name"=""}) -> ("Image Out"=w321:T1, "Fitted Circle (Find Circular Edge 1)"=w316:T6)  [unwired: 22 in, 1 out]
      n90 = call "KB-laser 计算同心度.vi"("小圆圆心"=w316, "大圆圆心"=w317) -> ("sqrt(x)"=w315:sgl)  [unwired: 9 in]
      n91 = call "KB-Laser 寻找內圆.vi"("旧ROI"=w320, "新圆心"=w316) -> ("ROI Descriptor"=w319:T2)  [unwired: 6 in, 3 out]
    }
    frame "Item14" {
      (unwired) 3
      n92 = call "Vision Assistant14"("Image In"=w352, "ROI Descriptor (Find Circular Edge 1)"=w349, "Options (Find Circular Edge 1)"=T5 {"Search  Direction"=0, "Edge Options"={"Edge Polarity"=1, "Kernel Size"=13, "Width"=13, "Minimum Edge Strength"=35.0, "Interpolation Type"=enum."Bilinear Fixed", "Data Processing Method"=enum."Average"}, "Show Search Area"=TRUE, "Show Search Lines"=FALSE, "Show Edges Found"=FALSE, "Show Result"=TRUE, "Search Area Color"=65280, "Search Lines Color"=255, "Edge Locations Color"=16776960, "Result Color"=16711680, "Overlay Group Name"=""}) -> ("Image Out"=w341:T1, "Fitted Circle (Find Circular Edge 1)"=w336:T6)  [unwired: 21 in, 2 out]
      n93 = call "KB-Laser move.vi"("Fitted Circle (Find Circular Edge 1)"=w336, "I roi"=w346, "O roi"=w351) -> ("O roi Out"=w350:T2)  [unwired: 7 in, 1 out]
      n94 = call "KB-CalNew4Point.vi"("矩形ROS 原始"=w348, "Fitted Circle (Find Circular Edge 1) New"=w336, "原始寻心点"=w349) -> ("矩形ROS new"=w347:string[])  [unwired: 8 in]
      n95 = call "KB-CalNewC.vi"("Outer Radius"=75, "I roi"=w346, "Fitted Circle (Find Circular Edge 1)"=w336) -> ("ROI Descriptor"=w340:T2)  [unwired: 8 in]
      n96 = call "Find inner11"("Image In"=w341, "ROI Descriptor (Find Circular Edge 1)"=w340, "Options (Find Circular Edge 1)"=T5 {"Search  Direction"=0, "Edge Options"={"Edge Polarity"=2, "Kernel Size"=3, "Width"=3, "Minimum Edge Strength"=1.0, "Interpolation Type"=enum."Bilinear Fixed", "Data Processing Method"=enum."Average"}, "Show Search Area"=TRUE, "Show Search Lines"=FALSE, "Show Edges Found"=FALSE, "Show Result"=TRUE, "Search Area Color"=65280, "Search Lines Color"=255, "Edge Locations Color"=16776960, "Result Color"=16711680, "Overlay Group Name"=""}) -> ("Image Out"=w337:T1, "Fitted Circle (Find Circular Edge 1)"=w335:T6)  [unwired: 22 in, 1 out]
      n97 = call "KB-laser 计算同心度.vi"("小圆圆心"=w335, "大圆圆心"=w336) -> ("sqrt(x)"=w334:sgl)  [unwired: 9 in]
      n98 = call "KB-Laser 寻找內圆.vi"("旧ROI"=w340, "新圆心"=w335) -> ("ROI Descriptor"=w339:T2)  [unwired: 6 in, 3 out]
    }
    frame "Item15" {
      n99 = call "Vision Assistant15"("Image In"=w372, "ROI Descriptor (Find Circular Edge 1)"=w369, "Options (Find Circular Edge 1)"=T5 {"Search  Direction"=0, "Edge Options"={"Edge Polarity"=1, "Kernel Size"=13, "Width"=13, "Minimum Edge Strength"=35.0, "Interpolation Type"=enum."Bilinear Fixed", "Data Processing Method"=enum."Average"}, "Show Search Area"=TRUE, "Show Search Lines"=FALSE, "Show Edges Found"=FALSE, "Show Result"=TRUE, "Search Area Color"=65280, "Search Lines Color"=255, "Edge Locations Color"=16776960, "Result Color"=16711680, "Overlay Group Name"=""}) -> ("Image Out"=w360:T1, "Fitted Circle (Find Circular Edge 1)"=w355:T6, "Matches (Geometric Matching 1)"=w363:T7[])  [unwired: 21 in, 1 out]
      n100 = call "KB-Laser move.vi"("Matches (Geometric Matching 1)"=w363, "Fitted Circle (Find Circular Edge 1)"=w355, "I roi"=w366, "O roi"=w371) -> ("O roi Out"=w370:T2)  [unwired: 6 in, 1 out]
      n101 = call "KB-CalNew4Point.vi"("矩形ROS 原始"=w368, "Fitted Circle (Find Circular Edge 1) New"=w355, "原始寻心点"=w369) -> ("矩形ROS new"=w367:string[])  [unwired: 8 in]
      n102 = call "KB-CalNewC.vi"("Matches (Geometric Matching 1)"=w363, "Outer Radius"=75, "I roi"=w366, "Fitted Circle (Find Circular Edge 1)"=w355) -> ("ROI Descriptor"=w358:T2)  [unwired: 7 in]
      n103 = call "Find inner12"("Image In"=w360, "ROI Descriptor (Find Circular Edge 1)"=w358, "Options (Find Circular Edge 1)"=T5 {"Search  Direction"=0, "Edge Options"={"Edge Polarity"=2, "Kernel Size"=3, "Width"=3, "Minimum Edge Strength"=1.0, "Interpolation Type"=enum."Bilinear Fixed", "Data Processing Method"=enum."Average"}, "Show Search Area"=TRUE, "Show Search Lines"=FALSE, "Show Edges Found"=FALSE, "Show Result"=TRUE, "Search Area Color"=65280, "Search Lines Color"=255, "Edge Locations Color"=16776960, "Result Color"=16711680, "Overlay Group Name"=""}) -> ("Image Out"=w359:T1, "Fitted Circle (Find Circular Edge 1)"=w354:T6)  [unwired: 22 in, 1 out]
      n104 = call "KB-laser 计算同心度.vi"("小圆圆心"=w354, "大圆圆心"=w355) -> ("sqrt(x)"=w353:sgl)  [unwired: 9 in]
      n105 = call "KB-Laser 寻找內圆.vi"("旧ROI"=w358, "新圆心"=w354) -> ("ROI Descriptor"=w357:T2)  [unwired: 6 in, 3 out]
    }
    frame "Item16" {
      (unwired) 3
      n106 = call "Vision Assistant16"("Image In"=w391, "ROI Descriptor (Find Circular Edge 1)"=w388, "Options (Find Circular Edge 1)"=T5 {"Search  Direction"=0, "Edge Options"={"Edge Polarity"=1, "Kernel Size"=13, "Width"=13, "Minimum Edge Strength"=35.0, "Interpolation Type"=enum."Bilinear Fixed", "Data Processing Method"=enum."Average"}, "Show Search Area"=TRUE, "Show Search Lines"=FALSE, "Show Edges Found"=FALSE, "Show Result"=TRUE, "Search Area Color"=65280, "Search Lines Color"=255, "Edge Locations Color"=16776960, "Result Color"=16711680, "Overlay Group Name"=""}) -> ("Image Out"=w380:T1, "Fitted Circle (Find Circular Edge 1)"=w375:T6)  [unwired: 21 in, 2 out]
      n107 = call "KB-Laser move.vi"("Fitted Circle (Find Circular Edge 1)"=w375, "I roi"=w385, "O roi"=w390) -> ("O roi Out"=w389:T2)  [unwired: 7 in, 1 out]
      n108 = call "KB-CalNew4Point.vi"("矩形ROS 原始"=w387, "Fitted Circle (Find Circular Edge 1) New"=w375, "原始寻心点"=w388) -> ("矩形ROS new"=w386:string[])  [unwired: 8 in]
      n109 = call "KB-CalNewC.vi"("Outer Radius"=75, "I roi"=w385, "Fitted Circle (Find Circular Edge 1)"=w375) -> ("ROI Descriptor"=w379:T2)  [unwired: 8 in]
      n110 = call "Find inner13"("Image In"=w380, "ROI Descriptor (Find Circular Edge 1)"=w379, "Options (Find Circular Edge 1)"=T5 {"Search  Direction"=0, "Edge Options"={"Edge Polarity"=2, "Kernel Size"=3, "Width"=3, "Minimum Edge Strength"=1.0, "Interpolation Type"=enum."Bilinear Fixed", "Data Processing Method"=enum."Average"}, "Show Search Area"=TRUE, "Show Search Lines"=FALSE, "Show Edges Found"=FALSE, "Show Result"=TRUE, "Search Area Color"=65280, "Search Lines Color"=255, "Edge Locations Color"=16776960, "Result Color"=16711680, "Overlay Group Name"=""}) -> ("Image Out"=w377:T1, "Fitted Circle (Find Circular Edge 1)"=w374:T6)  [unwired: 22 in, 1 out]
      n111 = call "KB-laser 计算同心度.vi"("小圆圆心"=w374, "大圆圆心"=w375) -> ("sqrt(x)"=w373:sgl)  [unwired: 9 in]
      n112 = call "KB-Laser 寻找內圆.vi"("旧ROI"=w379, "新圆心"=w374) -> ("ROI Descriptor"=w378:T2)  [unwired: 6 in, 3 out]
    }
    frame "Item17" {
      (unwired) 16
      n113 = call "Vision Assistant17"("Image In"=w410, "ROI Descriptor (Find Circular Edge 1)"=w407, "Options (Find Circular Edge 1)"=T5 {"Search  Direction"=0, "Edge Options"={"Edge Polarity"=1, "Kernel Size"=13, "Width"=13, "Minimum Edge Strength"=35.0, "Interpolation Type"=enum."Bilinear Fixed", "Data Processing Method"=enum."Average"}, "Show Search Area"=TRUE, "Show Search Lines"=FALSE, "Show Edges Found"=FALSE, "Show Result"=TRUE, "Search Area Color"=65280, "Search Lines Color"=255, "Edge Locations Color"=16776960, "Result Color"=16711680, "Overlay Group Name"=""}) -> ("Image Out"=w399:T1, "Fitted Circle (Find Circular Edge 1)"=w394:T6)  [unwired: 21 in, 2 out]
      n114 = call "KB-Laser move.vi"("Fitted Circle (Find Circular Edge 1)"=w394, "I roi"=w404, "O roi"=w409) -> ("O roi Out"=w408:T2)  [unwired: 7 in, 1 out]
      n115 = call "KB-CalNew4Point.vi"("矩形ROS 原始"=w406, "Fitted Circle (Find Circular Edge 1) New"=w394, "原始寻心点"=w407) -> ("矩形ROS new"=w405:string[])  [unwired: 8 in]
      n116 = call "KB-CalNewC.vi"("Outer Radius"=75, "I roi"=w404, "Fitted Circle (Find Circular Edge 1)"=w394) -> ("ROI Descriptor"=w398:T2)  [unwired: 8 in]
      n117 = call "Find inner14"("Image In"=w399, "ROI Descriptor (Find Circular Edge 1)"=w398, "Options (Find Circular Edge 1)"=T5 {"Search  Direction"=0, "Edge Options"={"Edge Polarity"=2, "Kernel Size"=3, "Width"=3, "Minimum Edge Strength"=1.0, "Interpolation Type"=enum."Bilinear Fixed", "Data Processing Method"=enum."Average"}, "Show Search Area"=TRUE, "Show Search Lines"=FALSE, "Show Edges Found"=FALSE, "Show Result"=TRUE, "Search Area Color"=65280, "Search Lines Color"=255, "Edge Locations Color"=16776960, "Result Color"=16711680, "Overlay Group Name"=""}) -> ("Image Out"=w395:T1, "Fitted Circle (Find Circular Edge 1)"=w393:T6)  [unwired: 22 in, 1 out]
      n118 = call "KB-laser 计算同心度.vi"("小圆圆心"=w393, "大圆圆心"=w394) -> ("sqrt(x)"=w392:sgl)  [unwired: 9 in]
      n119 = call "KB-Laser 寻找內圆.vi"("旧ROI"=w398, "新圆心"=w393) -> ("ROI Descriptor"=w397:T2)  [unwired: 6 in, 3 out]
    }
    frame "Item18" {
      (unwired) 16
      n120 = call "Vision Assistant18"("Image In"=w429, "ROI Descriptor (Find Circular Edge 1)"=w426, "Options (Find Circular Edge 1)"=T5 {"Search  Direction"=0, "Edge Options"={"Edge Polarity"=1, "Kernel Size"=13, "Width"=13, "Minimum Edge Strength"=35.0, "Interpolation Type"=enum."Bilinear Fixed", "Data Processing Method"=enum."Average"}, "Show Search Area"=TRUE, "Show Search Lines"=FALSE, "Show Edges Found"=FALSE, "Show Result"=TRUE, "Search Area Color"=65280, "Search Lines Color"=255, "Edge Locations Color"=16776960, "Result Color"=16711680, "Overlay Group Name"=""}) -> ("Image Out"=w418:T1, "Fitted Circle (Find Circular Edge 1)"=w413:T6)  [unwired: 21 in, 2 out]
      n121 = call "KB-Laser move.vi"("Fitted Circle (Find Circular Edge 1)"=w413, "I roi"=w423, "O roi"=w428) -> ("O roi Out"=w427:T2)  [unwired: 7 in, 1 out]
      n122 = call "KB-CalNew4Point.vi"("矩形ROS 原始"=w425, "Fitted Circle (Find Circular Edge 1) New"=w413, "原始寻心点"=w426) -> ("矩形ROS new"=w424:string[])  [unwired: 8 in]
      n123 = call "KB-CalNewC.vi"("Outer Radius"=75, "I roi"=w423, "Fitted Circle (Find Circular Edge 1)"=w413) -> ("ROI Descriptor"=w416:T2)  [unwired: 8 in]
      n124 = call "Find inner15"("Image In"=w418, "ROI Descriptor (Find Circular Edge 1)"=w416, "Options (Find Circular Edge 1)"=T5 {"Search  Direction"=0, "Edge Options"={"Edge Polarity"=2, "Kernel Size"=3, "Width"=3, "Minimum Edge Strength"=1.0, "Interpolation Type"=enum."Bilinear Fixed", "Data Processing Method"=enum."Average"}, "Show Search Area"=TRUE, "Show Search Lines"=FALSE, "Show Edges Found"=FALSE, "Show Result"=TRUE, "Search Area Color"=65280, "Search Lines Color"=255, "Edge Locations Color"=16776960, "Result Color"=16711680, "Overlay Group Name"=""}) -> ("Image Out"=w417:T1, "Fitted Circle (Find Circular Edge 1)"=w412:T6)  [unwired: 22 in, 1 out]
      n125 = call "KB-laser 计算同心度.vi"("小圆圆心"=w412, "大圆圆心"=w413) -> ("sqrt(x)"=w411:sgl)  [unwired: 9 in]
      n126 = call "KB-Laser 寻找內圆.vi"("旧ROI"=w416, "新圆心"=w412) -> ("ROI Descriptor"=w415:T2)  [unwired: 6 in, 3 out]
    }
    frame "Item19" {
      (unwired) 16
      n127 = call "Vision Assistant19"("Image In"=w448, "ROI Descriptor (Find Circular Edge 1)"=w445, "Options (Find Circular Edge 1)"=T5 {"Search  Direction"=0, "Edge Options"={"Edge Polarity"=1, "Kernel Size"=13, "Width"=13, "Minimum Edge Strength"=35.0, "Interpolation Type"=enum."Bilinear Fixed", "Data Processing Method"=enum."Average"}, "Show Search Area"=TRUE, "Show Search Lines"=FALSE, "Show Edges Found"=FALSE, "Show Result"=TRUE, "Search Area Color"=65280, "Search Lines Color"=255, "Edge Locations Color"=16776960, "Result Color"=16711680, "Overlay Group Name"=""}) -> ("Image Out"=w437:T1, "Fitted Circle (Find Circular Edge 1)"=w432:T6)  [unwired: 21 in, 2 out]
      n128 = call "KB-Laser move.vi"("Fitted Circle (Find Circular Edge 1)"=w432, "I roi"=w442, "O roi"=w447) -> ("O roi Out"=w446:T2)  [unwired: 7 in, 1 out]
      n129 = call "KB-CalNew4Point.vi"("矩形ROS 原始"=w444, "Fitted Circle (Find Circular Edge 1) New"=w432, "原始寻心点"=w445) -> ("矩形ROS new"=w443:string[])  [unwired: 8 in]
      n130 = call "KB-CalNewC.vi"("Outer Radius"=75, "I roi"=w442, "Fitted Circle (Find Circular Edge 1)"=w432) -> ("ROI Descriptor"=w435:T2)  [unwired: 8 in]
      n131 = call "Find inner16"("Image In"=w437, "ROI Descriptor (Find Circular Edge 1)"=w435, "Options (Find Circular Edge 1)"=T5 {"Search  Direction"=0, "Edge Options"={"Edge Polarity"=2, "Kernel Size"=3, "Width"=3, "Minimum Edge Strength"=1.0, "Interpolation Type"=enum."Bilinear Fixed", "Data Processing Method"=enum."Average"}, "Show Search Area"=TRUE, "Show Search Lines"=FALSE, "Show Edges Found"=FALSE, "Show Result"=TRUE, "Search Area Color"=65280, "Search Lines Color"=255, "Edge Locations Color"=16776960, "Result Color"=16711680, "Overlay Group Name"=""}) -> ("Image Out"=w436:T1, "Fitted Circle (Find Circular Edge 1)"=w431:T6)  [unwired: 22 in, 1 out]
      n132 = call "KB-laser 计算同心度.vi"("小圆圆心"=w431, "大圆圆心"=w432) -> ("sqrt(x)"=w430:sgl)  [unwired: 9 in]
      n133 = call "KB-Laser 寻找內圆.vi"("旧ROI"=w435, "新圆心"=w431) -> ("ROI Descriptor"=w434:T2)  [unwired: 6 in, 3 out]
    }
    frame "Item20" {
      (unwired) 16
      n134 = call "Vision Assistant20"("Image In"=w467, "ROI Descriptor (Find Circular Edge 1)"=w464, "Options (Find Circular Edge 1)"=T5 {"Search  Direction"=0, "Edge Options"={"Edge Polarity"=1, "Kernel Size"=13, "Width"=13, "Minimum Edge Strength"=35.0, "Interpolation Type"=enum."Bilinear Fixed", "Data Processing Method"=enum."Average"}, "Show Search Area"=TRUE, "Show Search Lines"=FALSE, "Show Edges Found"=FALSE, "Show Result"=TRUE, "Search Area Color"=65280, "Search Lines Color"=255, "Edge Locations Color"=16776960, "Result Color"=16711680, "Overlay Group Name"=""}) -> ("Image Out"=w456:T1, "Fitted Circle (Find Circular Edge 1)"=w451:T6)  [unwired: 21 in, 2 out]
      n135 = call "KB-Laser move.vi"("Fitted Circle (Find Circular Edge 1)"=w451, "I roi"=w461, "O roi"=w466) -> ("O roi Out"=w465:T2)  [unwired: 7 in, 1 out]
      n136 = call "KB-CalNew4Point.vi"("矩形ROS 原始"=w463, "Fitted Circle (Find Circular Edge 1) New"=w451, "原始寻心点"=w464) -> ("矩形ROS new"=w462:string[])  [unwired: 8 in]
      n137 = call "KB-CalNewC.vi"("Outer Radius"=75, "I roi"=w461, "Fitted Circle (Find Circular Edge 1)"=w451) -> ("ROI Descriptor"=w454:T2)  [unwired: 8 in]
      n138 = call "Find inner17"("Image In"=w456, "ROI Descriptor (Find Circular Edge 1)"=w454, "Options (Find Circular Edge 1)"=T5 {"Search  Direction"=0, "Edge Options"={"Edge Polarity"=2, "Kernel Size"=3, "Width"=3, "Minimum Edge Strength"=1.0, "Interpolation Type"=enum."Bilinear Fixed", "Data Processing Method"=enum."Average"}, "Show Search Area"=TRUE, "Show Search Lines"=FALSE, "Show Edges Found"=FALSE, "Show Result"=TRUE, "Search Area Color"=65280, "Search Lines Color"=255, "Edge Locations Color"=16776960, "Result Color"=16711680, "Overlay Group Name"=""}) -> ("Image Out"=w455:T1, "Fitted Circle (Find Circular Edge 1)"=w450:T6)  [unwired: 22 in, 1 out]
      n139 = call "KB-laser 计算同心度.vi"("小圆圆心"=w450, "大圆圆心"=w451) -> ("sqrt(x)"=w449:sgl)  [unwired: 9 in]
      n140 = call "KB-Laser 寻找內圆.vi"("旧ROI"=w454, "新圆心"=w450) -> ("ROI Descriptor"=w453:T2)  [unwired: 6 in, 3 out]
    }
    frame "Item21" {
      (unwired) 16
      n141 = call "Vision Assistant21"("Image In"=w486, "ROI Descriptor (Find Circular Edge 1)"=w483, "Options (Find Circular Edge 1)"=T5 {"Search  Direction"=0, "Edge Options"={"Edge Polarity"=1, "Kernel Size"=13, "Width"=13, "Minimum Edge Strength"=35.0, "Interpolation Type"=enum."Bilinear Fixed", "Data Processing Method"=enum."Average"}, "Show Search Area"=TRUE, "Show Search Lines"=FALSE, "Show Edges Found"=FALSE, "Show Result"=TRUE, "Search Area Color"=65280, "Search Lines Color"=255, "Edge Locations Color"=16776960, "Result Color"=16711680, "Overlay Group Name"=""}) -> ("Image Out"=w475:T1, "Fitted Circle (Find Circular Edge 1)"=w470:T6)  [unwired: 21 in, 2 out]
      n142 = call "KB-CalNew4Point.vi"("矩形ROS 原始"=w482, "Fitted Circle (Find Circular Edge 1) New"=w470, "原始寻心点"=w483) -> ("矩形ROS new"=w481:string[])  [unwired: 8 in]
      n143 = call "KB-Laser move.vi"("Fitted Circle (Find Circular Edge 1)"=w470, "I roi"=w480, "O roi"=w485) -> ("O roi Out"=w484:T2)  [unwired: 7 in, 1 out]
      n144 = call "KB-CalNewC.vi"("Outer Radius"=75, "I roi"=w480, "Fitted Circle (Find Circular Edge 1)"=w470) -> ("ROI Descriptor"=w473:T2)  [unwired: 8 in]
      n145 = call "Find inner18"("Image In"=w475, "ROI Descriptor (Find Circular Edge 1)"=w473, "Options (Find Circular Edge 1)"=T5 {"Search  Direction"=0, "Edge Options"={"Edge Polarity"=2, "Kernel Size"=3, "Width"=3, "Minimum Edge Strength"=1.0, "Interpolation Type"=enum."Bilinear Fixed", "Data Processing Method"=enum."Average"}, "Show Search Area"=TRUE, "Show Search Lines"=FALSE, "Show Edges Found"=FALSE, "Show Result"=TRUE, "Search Area Color"=65280, "Search Lines Color"=255, "Edge Locations Color"=16776960, "Result Color"=16711680, "Overlay Group Name"=""}) -> ("Image Out"=w474:T1, "Fitted Circle (Find Circular Edge 1)"=w469:T6)  [unwired: 22 in, 1 out]
      n146 = call "KB-laser 计算同心度.vi"("小圆圆心"=w469, "大圆圆心"=w470) -> ("sqrt(x)"=w468:sgl)  [unwired: 9 in]
      n147 = call "KB-Laser 寻找內圆.vi"("旧ROI"=w473, "新圆心"=w469) -> ("ROI Descriptor"=w472:T2)  [unwired: 6 in, 3 out]
    }
    frame "Item22" {
      n148 = call "Vision Assistant13"("Image In"=w494, "ROI Descriptor (Find Circular Edge 1)"=w493, "Options (Find Circular Edge 1)"=T5 {"Search  Direction"=0, "Edge Options"={"Edge Polarity"=1, "Kernel Size"=59, "Width"=33, "Minimum Edge Strength"=128.0, "Interpolation Type"=enum."Bilinear Fixed", "Data Processing Method"=enum."Average"}, "Show Search Area"=TRUE, "Show Search Lines"=FALSE, "Show Edges Found"=FALSE, "Show Result"=TRUE, "Search Area Color"=65280, "Search Lines Color"=255, "Edge Locations Color"=16776960, "Result Color"=16711680, "Overlay Group Name"=""}) -> ("Image Out"=w492:T1, "Fitted Circle (Find Circular Edge 1)"=w490:T6)  [unwired: 22 in, 1 out]
      n149 = call "KB-Laser move.vi"("Fitted Circle (Find Circular Edge 1)"=w490, "I roi"=w499, "O roi"=w502) -> ("O roi Out"=w501:T2)  [unwired: 7 in, 1 out]
      n150 = call "KB-CalNew4Point.vi"("矩形ROS 原始"=w497, "Fitted Circle (Find Circular Edge 1) New"=w490, "原始寻心点"=w493) -> ("矩形ROS new"=w500:string[])  [unwired: 8 in]
      n151 = call "KB-CalNewC.vi"("Outer Radius"=60, "I roi"=w499, "Fitted Circle (Find Circular Edge 1)"=w490) -> ("ROI Descriptor"=w498:T2)  [unwired: 8 in]
    }
    frame "Item23" {
      (unwired) 16
      n152 = call "Vision Assistant23"("Image In"=w517, "ROI Descriptor (Find Circular Edge 1)"=w514, "Options (Find Circular Edge 1)"=T5 {"Search  Direction"=0, "Edge Options"={"Edge Polarity"=1, "Kernel Size"=3, "Width"=3, "Minimum Edge Strength"=78.0, "Interpolation Type"=enum."Bilinear Fixed", "Data Processing Method"=enum."Average"}, "Show Search Area"=TRUE, "Show Search Lines"=FALSE, "Show Edges Found"=FALSE, "Show Result"=TRUE, "Search Area Color"=65280, "Search Lines Color"=255, "Edge Locations Color"=16776960, "Result Color"=16711680, "Overlay Group Name"=""}) -> ("Image Out"=w504:T1, "Fitted Circle (Find Circular Edge 1)"=w507:T6)  [unwired: 22 in, 1 out]
      n153 = call "KB-CalNew4Point.vi"("矩形ROS 原始"=w513, "Fitted Circle (Find Circular Edge 1) New"=w507, "原始寻心点"=w514) -> ("矩形ROS new"=w512:string[])  [unwired: 8 in]
      n154 = call "KB-Laser move.vi"("Fitted Circle (Find Circular Edge 1)"=w507, "I roi"=w511, "O roi"=w516) -> ("O roi Out"=w515:T2)  [unwired: 7 in, 1 out]
      n155 = call "KB-CalNewC.vi"("Outer Radius"=w506, "I roi"=w511, "Fitted Circle (Find Circular Edge 1)"=w507) -> ("ROI Descriptor"=w510:T2)  [unwired: 8 in]
    }
    frame "Item24" {
      (unwired) 16
      n156 = call "Vision Assistant24"("Image In"=w534, "ROI Descriptor (Find Circular Edge 1)"=w531, "Options (Find Circular Edge 1)"=T5 {"Search  Direction"=0, "Edge Options"={"Edge Polarity"=1, "Kernel Size"=9, "Width"=13, "Minimum Edge Strength"=10.0, "Interpolation Type"=enum."Bilinear Fixed", "Data Processing Method"=enum."Average"}, "Show Search Area"=TRUE, "Show Search Lines"=FALSE, "Show Edges Found"=FALSE, "Show Result"=TRUE, "Search Area Color"=65280, "Search Lines Color"=255, "Edge Locations Color"=16776960, "Result Color"=16711680, "Overlay Group Name"=""}) -> ("Image Out"=w522:T1, "Fitted Circle (Find Circular Edge 1)"=w524:T6, "Matches (Geometric Matching 1)"=w520:T7[])  [unwired: 21 in, 1 out]
      n157 = call "KB-Laser move.vi"("Matches (Geometric Matching 1)"=w520, "Fitted Circle (Find Circular Edge 1)"=w524, "I roi"=w528, "O roi"=w533) -> ("O roi Out"=w532:T2)  [unwired: 6 in, 1 out]
      n158 = call "KB-CalNew4Point.vi"("矩形ROS 原始"=w530, "Fitted Circle (Find Circular Edge 1) New"=w524, "原始寻心点"=w531) -> ("矩形ROS new"=w529:string[])  [unwired: 8 in]
      n159 = call "KB-新画十字线.vi"("数组"=w520, "输入图片"=w522) -> ("输出图片"=w521:T1)  [unwired: 8 in, 1 out]
      n160 = call "KB-CalNewC.vi"("Matches (Geometric Matching 1)"=w520, "Outer Radius"=w523, "I roi"=w528, "Fitted Circle (Find Circular Edge 1)"=w524) -> ("ROI Descriptor"=w527:T2)  [unwired: 7 in]
    }
    frame "Item25" {
      (unwired) 16
      n161 = call "Vision Assistant25"("Image In"=w551, "ROI Descriptor (Find Circular Edge 1)"=w548, "Options (Find Circular Edge 1)"=T5 {"Search  Direction"=0, "Edge Options"={"Edge Polarity"=1, "Kernel Size"=3, "Width"=3, "Minimum Edge Strength"=10.0, "Interpolation Type"=enum."Bilinear Fixed", "Data Processing Method"=enum."Average"}, "Show Search Area"=TRUE, "Show Search Lines"=FALSE, "Show Edges Found"=FALSE, "Show Result"=TRUE, "Search Area Color"=65280, "Search Lines Color"=255, "Edge Locations Color"=16776960, "Result Color"=16711680, "Overlay Group Name"=""}) -> ("Image Out"=w539:T1, "Fitted Circle (Find Circular Edge 1)"=w541:T6, "Matches (Geometric Matching 1)"=w537:T7[])  [unwired: 21 in, 1 out]
      n162 = call "KB-CalNew4Point.vi"("矩形ROS 原始"=w547, "Fitted Circle (Find Circular Edge 1) New"=w541, "原始寻心点"=w548) -> ("矩形ROS new"=w546:string[])  [unwired: 8 in]
      n163 = call "KB-Laser move.vi"("Matches (Geometric Matching 1)"=w537, "Fitted Circle (Find Circular Edge 1)"=w541, "I roi"=w545, "O roi"=w550) -> ("O roi Out"=w549:T2)  [unwired: 6 in, 1 out]
      n164 = call "KB-新画十字线.vi"("数组"=w537, "输入图片"=w539) -> ("输出图片"=w538:T1)  [unwired: 8 in, 1 out]
      n165 = call "KB-CalNewC.vi"("Matches (Geometric Matching 1)"=w537, "Outer Radius"=w540, "I roi"=w545, "Fitted Circle (Find Circular Edge 1)"=w541) -> ("ROI Descriptor"=w544:T2)  [unwired: 7 in]
    }
    frame "Item26" {
      (unwired) 16
      n166 = call "Vision Assistant26"("Image In"=w568, "ROI Descriptor (Find Circular Edge 1)"=w565, "Options (Find Circular Edge 1)"=T5 {"Search  Direction"=0, "Edge Options"={"Edge Polarity"=1, "Kernel Size"=9, "Width"=7, "Minimum Edge Strength"=10.0, "Interpolation Type"=enum."Bilinear Fixed", "Data Processing Method"=enum."Average"}, "Show Search Area"=TRUE, "Show Search Lines"=FALSE, "Show Edges Found"=FALSE, "Show Result"=TRUE, "Search Area Color"=65280, "Search Lines Color"=255, "Edge Locations Color"=16776960, "Result Color"=16711680, "Overlay Group Name"=""}) -> ("Image Out"=w556:T1, "Fitted Circle (Find Circular Edge 1)"=w558:T6, "Matches (Geometric Matching 1)"=w554:T7[])  [unwired: 21 in, 1 out]
      n167 = call "KB-CalNew4Point.vi"("矩形ROS 原始"=w564, "Fitted Circle (Find Circular Edge 1) New"=w558, "原始寻心点"=w565) -> ("矩形ROS new"=w563:string[])  [unwired: 8 in]
      n168 = call "KB-Laser move.vi"("Matches (Geometric Matching 1)"=w554, "Fitted Circle (Find Circular Edge 1)"=w558, "I roi"=w562, "O roi"=w567) -> ("O roi Out"=w566:T2)  [unwired: 6 in, 1 out]
      n169 = call "KB-新画十字线.vi"("数组"=w554, "输入图片"=w556) -> ("输出图片"=w555:T1)  [unwired: 8 in, 1 out]
      n170 = call "KB-CalNewC.vi"("Matches (Geometric Matching 1)"=w554, "Outer Radius"=w557, "I roi"=w562, "Fitted Circle (Find Circular Edge 1)"=w558) -> ("ROI Descriptor"=w561:T2)  [unwired: 7 in]
    }
    frame "Item27" {
      (unwired) 16
      n171 = call "Vision Assistant27"("Image In"=w585, "ROI Descriptor (Find Circular Edge 1)"=w582, "Options (Find Circular Edge 1)"=T5 {"Search  Direction"=0, "Edge Options"={"Edge Polarity"=1, "Kernel Size"=13, "Width"=13, "Minimum Edge Strength"=100.0, "Interpolation Type"=enum."Bilinear Fixed", "Data Processing Method"=enum."Average"}, "Show Search Area"=TRUE, "Show Search Lines"=FALSE, "Show Edges Found"=FALSE, "Show Result"=TRUE, "Search Area Color"=65280, "Search Lines Color"=255, "Edge Locations Color"=16776960, "Result Color"=16711680, "Overlay Group Name"=""}) -> ("Image Out"=w573:T1, "Fitted Circle (Find Circular Edge 1)"=w575:T6, "Matches (Geometric Matching 1)"=w571:T7[])  [unwired: 21 in, 1 out]
      n172 = call "KB-Laser move.vi"("Matches (Geometric Matching 1)"=w571, "Fitted Circle (Find Circular Edge 1)"=w575, "I roi"=w579, "O roi"=w584) -> ("O roi Out"=w583:T2)  [unwired: 6 in, 1 out]
      n173 = call "KB-CalNew4Point.vi"("矩形ROS 原始"=w581, "Fitted Circle (Find Circular Edge 1) New"=w575, "原始寻心点"=w582) -> ("矩形ROS new"=w580:string[])  [unwired: 8 in]
      n174 = call "KB-新画十字线.vi"("数组"=w571, "输入图片"=w573) -> ("输出图片"=w572:T1)  [unwired: 8 in, 1 out]
      n175 = call "KB-CalNewC.vi"("Matches (Geometric Matching 1)"=w571, "Outer Radius"=w574, "I roi"=w579, "Fitted Circle (Find Circular Edge 1)"=w575) -> ("ROI Descriptor"=w578:T2)  [unwired: 7 in]
    }
    frame "Item28" {
      (unwired) 16
      n176 = call "Vision Assistant28"("Image In"=w592, "ROI Descriptor (Find Circular Edge 1)"=w600, "Options (Find Circular Edge 1)"=T5 {"Search  Direction"=0, "Edge Options"={"Edge Polarity"=1, "Kernel Size"=13, "Width"=13, "Minimum Edge Strength"=5.0, "Interpolation Type"=enum."Bilinear Fixed", "Data Processing Method"=enum."Average"}, "Show Search Area"=TRUE, "Show Search Lines"=FALSE, "Show Edges Found"=FALSE, "Show Result"=TRUE, "Search Area Color"=65280, "Search Lines Color"=255, "Edge Locations Color"=16776960, "Result Color"=16711680, "Overlay Group Name"=""}) -> ("Image Out"=w590:T1, "Fitted Circle (Find Circular Edge 1)"=w593:T6, "Matches (Geometric Matching 1)"=w588:T7[])  [unwired: 21 in, 1 out]
      n177 = call "KB-CalNew4Point.vi"("矩形ROS 原始"=w599, "Fitted Circle (Find Circular Edge 1) New"=w593, "原始寻心点"=w600) -> ("矩形ROS new"=w598:string[])  [unwired: 8 in]
      n178 = call "KB-Laser move.vi"("Matches (Geometric Matching 1)"=w588, "Fitted Circle (Find Circular Edge 1)"=w593, "I roi"=w597, "O roi"=w602) -> ("O roi Out"=w601:T2)  [unwired: 6 in, 1 out]
      n179 = call "KB-新画十字线.vi"("数组"=w588, "输入图片"=w590) -> ("输出图片"=w589:T1)  [unwired: 8 in, 1 out]
      n180 = call "KB-CalNewC.vi"("Matches (Geometric Matching 1)"=w588, "Outer Radius"=w591, "I roi"=w597, "Fitted Circle (Find Circular Edge 1)"=w593) -> ("ROI Descriptor"=w596:T2)  [unwired: 7 in]
    }
    frame "Item29" {
      (unwired) 16
      n181 = call "Vision Assistant29"("Image In"=w619, "ROI Descriptor (Find Circular Edge 1)"=w616, "Options (Find Circular Edge 1)"=T5 {"Search  Direction"=0, "Edge Options"={"Edge Polarity"=1, "Kernel Size"=13, "Width"=13, "Minimum Edge Strength"=63.0, "Interpolation Type"=enum."Bilinear Fixed", "Data Processing Method"=enum."Average"}, "Show Search Area"=TRUE, "Show Search Lines"=FALSE, "Show Edges Found"=FALSE, "Show Result"=TRUE, "Search Area Color"=65280, "Search Lines Color"=255, "Edge Locations Color"=16776960, "Result Color"=16711680, "Overlay Group Name"=""}) -> ("Image Out"=w607:T1, "Fitted Circle (Find Circular Edge 1)"=w609:T6, "Matches (Geometric Matching 1)"=w605:T7[])  [unwired: 21 in, 1 out]
      n182 = call "KB-Laser move.vi"("Matches (Geometric Matching 1)"=w605, "Fitted Circle (Find Circular Edge 1)"=w609, "I roi"=w613, "O roi"=w618) -> ("O roi Out"=w617:T2)  [unwired: 6 in, 1 out]
      n183 = call "KB-CalNew4Point.vi"("矩形ROS 原始"=w615, "Fitted Circle (Find Circular Edge 1) New"=w609, "原始寻心点"=w616) -> ("矩形ROS new"=w614:string[])  [unwired: 8 in]
      n184 = call "KB-新画十字线.vi"("数组"=w605, "输入图片"=w607) -> ("输出图片"=w606:T1)  [unwired: 8 in, 1 out]
      n185 = call "KB-CalNewC.vi"("Matches (Geometric Matching 1)"=w605, "Outer Radius"=w608, "I roi"=w613, "Fitted Circle (Find Circular Edge 1)"=w609) -> ("ROI Descriptor"=w612:T2)  [unwired: 7 in]
    }
    frame "Item30" {
      (unwired) 16
      n186 = call "Vision Assistant30"("Image In"=w637, "ROI Descriptor (Find Circular Edge 1)"=w634, "Options (Find Circular Edge 1)"=T5 {"Search  Direction"=0, "Edge Options"={"Edge Polarity"=1, "Kernel Size"=3, "Width"=1, "Minimum Edge Strength"=12.0, "Interpolation Type"=enum."Bilinear Fixed", "Data Processing Method"=enum."Average"}, "Show Search Area"=TRUE, "Show Search Lines"=FALSE, "Show Edges Found"=FALSE, "Show Result"=TRUE, "Search Area Color"=65280, "Search Lines Color"=255, "Edge Locations Color"=16776960, "Result Color"=16711680, "Overlay Group Name"=""}) -> ("Image Out"=w626:T1, "Fitted Circle (Find Circular Edge 1)"=w621:T6, "Matches (Geometric Matching 1)"=w624:T7[])  [unwired: 21 in, 1 out]
      n187 = call "KB-Laser move.vi"("Matches (Geometric Matching 1)"=w624, "Fitted Circle (Find Circular Edge 1)"=w621, "I roi"=w631, "O roi"=w636) -> ("O roi Out"=w635:T2)  [unwired: 6 in, 1 out]
      n188 = call "KB-CalNew4Point.vi"("矩形ROS 原始"=w633, "Fitted Circle (Find Circular Edge 1) New"=w621, "原始寻心点"=w634) -> ("矩形ROS new"=w632:string[])  [unwired: 8 in]
      n189 = call "KB-新画十字线.vi"("数组"=w624, "输入图片"=w626) -> ("Position"=w622:cluster{"x":sgl, "y":sgl}, "输出图片"=w625:T1)  [unwired: 8 in]
      n190 = call "KB-CalNewC.vi"("Matches (Geometric Matching 1)"=w624, "Outer Radius"=w627, "I roi"=w631, "Fitted Circle (Find Circular Edge 1)"=w621) -> ("ROI Descriptor"=w630:T2)  [unwired: 7 in]
    }
    frame "Item31" {
      (unwired) 16
      n191 = call "Vision Assistant31"("Image In"=w655, "ROI Descriptor (Find Circular Edge 1)"=w651, "Options (Find Circular Edge 1)"=T5 {"Search  Direction"=0, "Edge Options"={"Edge Polarity"=1, "Kernel Size"=17, "Width"=13, "Minimum Edge Strength"=20.0, "Interpolation Type"=enum."Bilinear Fixed", "Data Processing Method"=enum."Average"}, "Show Search Area"=TRUE, "Show Search Lines"=FALSE, "Show Edges Found"=FALSE, "Show Result"=TRUE, "Search Area Color"=65280, "Search Lines Color"=255, "Edge Locations Color"=16776960, "Result Color"=16711680, "Overlay Group Name"=""}) -> ("Image Out"=w643:T1, "Fitted Circle (Find Circular Edge 1)"=w644:T6, "Matches (Geometric Matching 1)"=w641:T7[], "error out"=w652:errorcluster)  [unwired: 21 in]
      n192 = call "KB-CalNew4Point.vi"("矩形ROS 原始"=w650, "Fitted Circle (Find Circular Edge 1) New"=w644, "原始寻心点"=w651) -> ("矩形ROS new"=w649:string[])  [unwired: 8 in]
      n193 = call "KB-Laser move.vi"("Matches (Geometric Matching 1)"=w641, "Fitted Circle (Find Circular Edge 1)"=w644, "I roi"=w648, "O roi"=w654) -> ("O roi Out"=w653:T2)  [unwired: 6 in, 1 out]
      n194 = call "KB-新画十字线.vi"("数组"=w641, "输入图片"=w643) -> ("输出图片"=w642:T1)  [unwired: 8 in, 1 out]
      n195 = call "KB-CalNewC.vi"("Matches (Geometric Matching 1)"=w641, "Outer Radius"=w640, "I roi"=w648, "Fitted Circle (Find Circular Edge 1)"=w644) -> ("ROI Descriptor"=w647:T2)  [unwired: 7 in]
    }
  }
  "Image Baser" <- w24
  "Image Baser 2" <- w24
  "矩形ROS new" <- w33
  "同心度" <- w8
  n196 = Decimal String To Number(string=w33) -> (number=w32:i32[])  [unwired: 2 in, 1 out]
  n197 = call "IMAQ Copy"("error in (no error)"=w48, "Image Dst"="Image  input  copy", "Image Src"=w24) -> ()  [unwired: 3 in, 2 out]
  n198 = Index Array(array=w32, index #1=0 ("索引")) -> (element #1=w28:i32, element #2=w27:i32)  [unwired: 1 in]
  n199 = Index Array(array=w25, index (row)=w27, index (col)=w28) -> (element=w30:dbl)
  n200 = call "KB-CalOffsetAndFlatness.vi"("Image In"=w24, "ROI Descriptor"=w22, "数值 2"="数值 2", "Row Select Laser"="Row Select Laser", "y"="y", "Src Data"=w23, "ROI  小圆"=w20, "数值"=w10) -> ("x-y"=→"x-y":dbl, "内外高低差-内部高到底差"=w37:dbl[], "外环平均高度值"=w15:dbl, "子数组 2"=→"内外3D":dbl[][], "内环3D"=→"内环3D":dbl[][], "外环3D"=→"外环3D":dbl[][])  [unwired: 5 in, 1 out]
  n201 = Subtract(x=w15, y=w30) -> (x-y=w12:dbl)
  n202 = case shown="\"Item22\"" "Row Select Laser" {
    tunnel: w12 -> [w658 w661]
    tunnel: [w657 w660] -> w11
    tunnel: "raoto1" -> [w656 w659]
    frame "假", Default {
      n203 = Multiply(x=w658, y=w656) -> (x*y=w657:dbl)
    }
    frame "Item22" {
      n204 = Multiply(x=w661, y=w659) -> (x*y=w660:dbl)
    }
  }
  n205 = Number To Fractional String(number=w37, precision (6)=i16 3 ("精度(6)")) -> (F-format string=w35:string[])  [unwired: 2 in]
  n206 = Index Array(array=w35) -> (element #1=w2:string, element #2=w34:string)  [unwired: 2 in]
  n207 = Number To Fractional String(number=w8, precision (6)=i16 3 ("精度(6)")) -> (F-format string=w7:string)  [unwired: 2 in]
  n208 = Equal?(x=w2, y="NaN") -> (x = y?=w3:bool)
  n209 = case shown="假" w3 {
    tunnel: w2 -> [w662 _]
    tunnel: [w662 w663] -> w1
    frame False {
    }
    frame True {
      n210 = Random Number (0-1) "随机数(0-1)"() -> (number: 0 to 1=w669:dbl)
      n211 = Multiply(x=w669, y=2) -> (x*y=w667:dbl)
      n212 = Divide(x=w667, y=10.0) -> (x/y=w664:dbl)
      n213 = Number To Fractional String(number=w664, precision (6)=i16 3 ("精度(6)")) -> (F-format string=w663:string)  [unwired: 2 in]
    }
  }
  n214 = Number To Fractional String(number=w11, precision (6)=i16 3 ("精度(6)")) -> (F-format string=w29:string)  [unwired: 2 in]
  n215 = case shown="21..30" w41 {
    tunnel: w1 -> [w672 w675 w678 w681 w684 w687 _ _ _ _ w694 w697]
    tunnel: w34 -> [w671 w674 w677 w680 w683 w686 _ _ _ _ w693 w696]
    tunnel: [w672 w675 w678 w681 w684 w687 w688 w689 w690 w691 w694 w697] -> w40
    tunnel: [w671 w674 w677 w680 w683 w686 w688 w689 w690 w691 w693 w696] -> w39
    tunnel: ["Null" "Null" "Null" "Null" "Null" "Null" w688 w689 w690 w691 "Null" w695] -> w38
    tunnel: w29 -> [_ _ _ _ _ _ _ _ _ _ _ w695]
    frame 0, Default {
    }
    frame 1 {
    }
    frame 2 {
    }
    frame 3 {
    }
    frame 4 {
    }
    frame 5 {
    }
    frame 6 {
      w688 = "Null"
    }
    frame 7 {
      w689 = "Null"
    }
    frame 8 {
      w690 = "Null"
    }
    frame 9 {
      w691 = "Null"
    }
    frame 10..20 {
    }
    frame 21..30 {
    }
  }
  n216 = Build Array(w40, w39, w38, w7) -> (→"Result Array":string[])
  "Row Select Laser 2" <- "Row Select Laser"
